vi "Steuerprogramm_ECD-HorstTest.vi"() -> ()   [LabVIEW 2017]
uses:
  <vilib>/FPGAPlugInAG/cRIO-9035/niLvFpga_Close_cRIO-9035.vi
  <vilib>/rvi/errors/niLvFpgaAdjustHostInterfaceError.vi
  <vilib>/Utility/error.llb/Error Cluster From Error Code.vi
  GVRefStrom.vi
  gvbooleschRT.vi
  GVMethodenwechsel.vi
  GVZeitenZyklen.vi
  GVaktuelleTDMS.vi
  GVChroms.vi
  GVMetavariablen.vi
  GVMWHorst.vi
  GVVentilposition.vi
  GVHK1Hz.vi
  GVZwangs.vi
  GVZwangsMPV.vi
  GVTrapsMachs.vi
  GVECDs.vi
  GVAIs.vi
  GVHeizenLH.vi
  GVHorstSP.vi
  GVProbenvol.vi
  <vilib>/rvi/interface/nirviCloseFPGA/nirviCloseFPGA.xnode
  FPGA Bitfiles/HAGAR-VECD_FPGATarget_FPGA-ProgrammECD_WS++LmW9gGg.lvbitx
  FPGA-Programm_ECD.vi
  <vilib>/rvi/interface/nirviReadWriteControl/nirviReadWriteControl.xnode
  <vilib>/rvi/interface/nirviMethod/nirviMethod.xnode
  <vilib>/rvi/errors/niLvFpgaMergeErrorWithErrorCode.vi
  <vilib>/FPGAPlugInAG/cRIO-9035/niLvFpga_WriteFifo_cRIO-9035.vi
  NiFpgaLv.dll
panel:
  out "Fehler ECD1alt":errorcluster caption="Fehler (Ausgang)"
  in  "Methode speichern":bool
  out "ZyklusNummernGesamt":i32[](array[numeric])
  in  "veränderte Methode benutzen":bool
  in  "Methode verändern":bool
  out "ZyklusNummern":i32[](array[numeric])
  out "Big Ben, Methodenzeit, Zykluszeit0, Zykluszeit1, Zykluszeit2A, Zykluszeit2B":i32[](array[numeric])
  in  "global stop RT":bool
  in  "Methode":i32(ring) items=["Bedingsmethode", "Startmethode", "Meßmodus", "Shut-up-Methode", "Test", "HAG2 1/2", "Startmethode", "HAG2 1/2 Aufwärmen", "LicorDruckProfil1", "LicorDruckProfil2", "LicorDruckProfil0", "LicorDruckProfil3"]
  in  "Registerkarte":T1(tab)
  out "SHOK?":bool[](array[boolean])
  out "schnelle Heizungen":string[](array[string])
  out "schnelle Heizungen":dbl[](array[numeric])
  out "HorstOK?":bool[](array[boolean])
  out "AIs3OK?":bool[](array[boolean])
  out "AIs1OK?":bool[](array[boolean])
  out "AIs1":dbl[](array[numeric])
  out "AIs1":string[](array[string])
  out "AIs2":string[](array[string])
  out "AIs3":string[](array[string])
  out "AIs2":dbl[](array[numeric])
  out "AIs3":dbl[](array[numeric])
  out "Metavariablen":string[](array[string])
  out "Metavariablen":dbl[](array[numeric])
  out "MWHorst":dbl[](array[numeric])
  out "HorstRegler":string[](array[string])
  out "AIs2OK?":bool[](array[boolean])
  out "Ventilposition":i32=1 min=1 max=6 step=1
  out "MVOK?":bool[](array[boolean])
  in  "MV-Vorgaben":dbl[](array[numeric])
  in  "MV-Festhalten":bool[](array[boolean])
  in  "LH-Gruppe":bool[](array[boolean])=[FALSE, FALSE, FALSE, FALSE, FALSE, FALSE, FALSE, FALSE, FALSE, FALSE, FALSE, FALSE]
  out "LangsameHeizungen":string[](array[string])
  out "Housekeeping1":cluster{dbl[], dbl[]}(graph)
  in  "Zeitachse1":i32(ring)=1 items=["Zykluszeit [s] Mod0", "Zykluszeit [s] Mod1", "Zykluszeit [s] Mod2A", "Zykluszeit [s] Mod2B"]
  in  "dargestellte Größe 1":i32(ring)=1 items=["T1-Trap1 [°C]", "T1-Trap2 [°C]", "T1-StirlingKühlkopf [°C]", "T1-PreCol1 [°C]", "T1-PreCol2 [°C]", "T1-MainCol1a [°C]", "T1-MainCol1b [°C]", "T1-MainCol2a [°C]", "T1-MainCol2b [°C]", "T1-Bronkhorst1a [°C]", "T1-Bronkhorst1b [°C]", "T1-Bronkhorst2a [°C]", "T1-Bronkhorst2b [°C]", "T1-2Pos1B [°C]", "T1-Spare9", "T1-2Pos1A [°C]", "T1-Spare10", "T1-TurboPump [°C]", "T1-StirlingPlatine [°C]", "T1-Spare5", "T1-Spare6", "T1-Spare7", "T1-Inlet [°C]", "F1-MFM1", "F1-MFM0D [mL]", "P1-HeliumHP [bara]", "P1-HeliumLP [bara]", "P1-PumpVordruck [mbara]", "TurboSpeed", "I1-MS-AC [A]", "I1-Trap1 [A]", "I1-Trap2 [A]", "T2-ECD1a", "T2-ECD1b", "T2-ECD2a", "T2-ECD2b", "T2-Col1a", "T2-Col1b", "T2-Col2a", "T2-Col2b", "T2-Spare1", "T2-Spare2", "T2-Oven_a", "T2-Oven_b", "T2-Spare3", "T2-Spare4", "T2-Spare5", "F2-MFM0", "F2-MFM2A", "F2-MFM2B", "P2-N2O_HP", "P2-N2O_LP", "P2-CO2_HP", "P2-CO2_LP", "AI-Spare1", "FL-MFM1000mL", "AI-Spare3", "AI-Spare4", "StirlingAlarm", "StirlingEmerg.", "AI-Spare7", "AI-Spare8", "AI-Spare9", "FL-MFM30mL", "T0-DC/DC5", "I0-24V_M0", "I0-48V_M1", "I0-24V_M1", "I0-28V_M2", "T0-Spare3", "T0-Spare2", "T0-Spare4", "T0-DC/DC7", "I0-20V_Laptop", "I0-28V_M1", "I0-24V_M2", "I0-12V_Licor", "T0-Spare1", "T0-Drier", "T0-Spare5", "F0-MFM0A [L]", "TL-Licor_a", "P0-Span-HP", "P0-spare1", "P0-Stickstoff-LP", "P0-Helium-LP", "P0-Cal-HP", "P0-P9Tavco[bar]", "F0-MFM0B [L]", "TL-Licor_b", "P0-Span-LP", "P0-spare2", "P0-Stickstoff-HP", "P0-Helium-HP", "P0-Cal-LP", "F0-MFM3", "TemperaturTrap1[°C]", "TemperaturTrap2[°C]", "TemperaturPreMach1[°C]", "TemperaturPreMach2[°C]", "TemperaturMainMach1[°C]", "TemperaturMainMach2[°C]", "PrC0 [bara]", "PrC0-Licor [bara]", "PrC1-Säule1 [bara]", "PrC1-Säule2 [bara]", "MFC1-Sample [ml/min]", "PrC1-BackFlush1 [bara]", "PrC1-BackFlush2 [bara]", "MFC1-Reaktant [l/min]", "MFC2A[ml/min]", "MFC2B[ml/min]", "MFC2C[ul/min]", "PrC2A[bara]", "MFC2D[ml/min]", "MFC2E[ml/min]", "PrC2B[bara]"]
  out "Housekeeping2":cluster{dbl[], dbl[]}(graph)
  in  "Zeitachse2":i32(ring)=1 items=["Zykluszeit [s] Mod0", "Zykluszeit [s] Mod1", "Zykluszeit [s] Mod2A", "Zykluszeit [s] Mod2B"]
  in  "dargestellte Größe 2":i32(ring)=1 items=["T1-Trap1 [°C]", "T1-Trap2 [°C]", "T1-StirlingKühlkopf [°C]", "T1-PreCol1 [°C]", "T1-PreCol2 [°C]", "T1-MainCol1a [°C]", "T1-MainCol1b [°C]", "T1-MainCol2a [°C]", "T1-MainCol2b [°C]", "T1-Bronkhorst1a [°C]", "T1-Bronkhorst1b [°C]", "T1-Bronkhorst2a [°C]", "T1-Bronkhorst2b [°C]", "T1-2Pos1B [°C]", "T1-Spare9", "T1-2Pos1A [°C]", "T1-Spare10", "T1-TurboPump [°C]", "T1-StirlingPlatine [°C]", "T1-Spare5", "T1-Spare6", "T1-Spare7", "T1-Inlet [°C]", "F1-MFM1", "F1-MFM0D [mL]", "P1-HeliumHP [bara]", "P1-HeliumLP [bara]", "P1-PumpVordruck [mbara]", "TurboSpeed", "I1-MS-AC [A]", "I1-Trap1 [A]", "I1-Trap2 [A]", "T2-ECD1a", "T2-ECD1b", "T2-ECD2a", "T2-ECD2b", "T2-Col1a", "T2-Col1b", "T2-Col2a", "T2-Col2b", "T2-Spare1", "T2-Spare2", "T2-Oven_a", "T2-Oven_b", "T2-Spare3", "T2-Spare4", "T2-Spare5", "F2-MFM0", "F2-MFM2A", "F2-MFM2B", "P2-N2O_HP", "P2-N2O_LP", "P2-CO2_HP", "P2-CO2_LP", "AI-Spare1", "FL-MFM1000mL", "AI-Spare3", "AI-Spare4", "StirlingAlarm", "StirlingEmerg.", "AI-Spare7", "AI-Spare8", "AI-Spare9", "FL-MFM30mL", "T0-DC/DC5", "I0-24V_M0", "I0-48V_M1", "I0-24V_M1", "I0-28V_M2", "T0-Spare3", "T0-Spare2", "T0-Spare4", "T0-DC/DC7", "I0-20V_Laptop", "I0-28V_M1", "I0-24V_M2", "I0-12V_Licor", "T0-Spare1", "T0-Drier", "T0-Spare5", "F0-MFM0A [L]", "TL-Licor_a", "P0-Span-HP", "P0-spare1", "P0-Stickstoff-LP", "P0-Helium-LP", "P0-Cal-HP", "P0-P9Tavco[bar]", "F0-MFM0B [L]", "TL-Licor_b", "P0-Span-LP", "P0-spare2", "P0-Stickstoff-HP", "P0-Helium-HP", "P0-Cal-LP", "F0-MFM3", "TemperaturTrap1[°C]", "TemperaturTrap2[°C]", "TemperaturPreMach1[°C]", "TemperaturPreMach2[°C]", "TemperaturMainMach1[°C]", "TemperaturMainMach2[°C]", "PrC0 [bara]", "PrC0-Licor [bara]", "PrC1-Säule1 [bara]", "PrC1-Säule2 [bara]", "MFC1-Sample [ml/min]", "PrC1-BackFlush1 [bara]", "PrC1-BackFlush2 [bara]", "MFC1-Reaktant [l/min]", "MFC2A[ml/min]", "MFC2B[ml/min]", "MFC2C[ul/min]", "PrC2A[bara]", "MFC2D[ml/min]", "MFC2E[ml/min]", "PrC2B[bara]"]
  out "Detektor 2":cluster{dbl[], dbl[]}[](graph)
  in  "Detektor":i32(ring) items=["ECD1", "ECD2"]
  in  "HK1YMin":dbl
  in  "HK1YMax":dbl=100.0
  in  "HK2YMin":dbl
  in  "HK2YMax":dbl=100.0
  in  "DetYMin":dbl
  in  "DetYMax":dbl=100.0
  in  "RefStromECD2":i16=2000 min=0 max=2500 step=1
  in  "RefStromECD1":i16=2000 min=0 max=2500 step=1
  out "schnelleAnzeige":cluster{dbl[], dbl[]}(graph)
  in  "TafelWischen!":bool
  in  "dargestellte Größe 3":i32(ring)=1 items=["TemperaturTrap1[°C]", "TemperaturTrap2[°C]", "TemperaturPreMach1[°C]", "TemperaturPreMach2[°C]", "TemperaturMainMach1[°C]", "TemperaturMainMach2[°C]", "PrC0 [bara]", "PrC0-Licor [bara]", "PrC1-Säule1 [bara]", "PrC1-Säule2 [bara]", "MFC1-Sample [ml/min]", "PrC1-BackFlush1 [bara]", "PrC1-BackFlush2 [bara]", "MFC1-Reaktant [l/min]", "MFC2A[ml/min]", "MFC2B[ml/min]", "MFC2C[ul/min]", "PrC2A[bara]", "MFC2D[ml/min]", "MFC2E[ml/min]", "PrC2B[bara]"]
  in  "An/Aus":bool
  out "TDMSwriteECD":errorcluster
  out "AIsFIFOread":errorcluster
  out "MWTrapsMachs":errorcluster
  out "TDMSwriteHK":errorcluster
  out "TDMScloseHK":errorcluster
  out "TDMSopenHK":errorcluster
  out "TDMScloseECD2":errorcluster
  out "TDMSopenECD2":errorcluster
  out "TDMScloseECD1":errorcluster
  out "TDMSopenECD1":errorcluster
  out "SerielleKomm.":errorcluster
  out "LH":errorcluster
  out "Zyklus":errorcluster
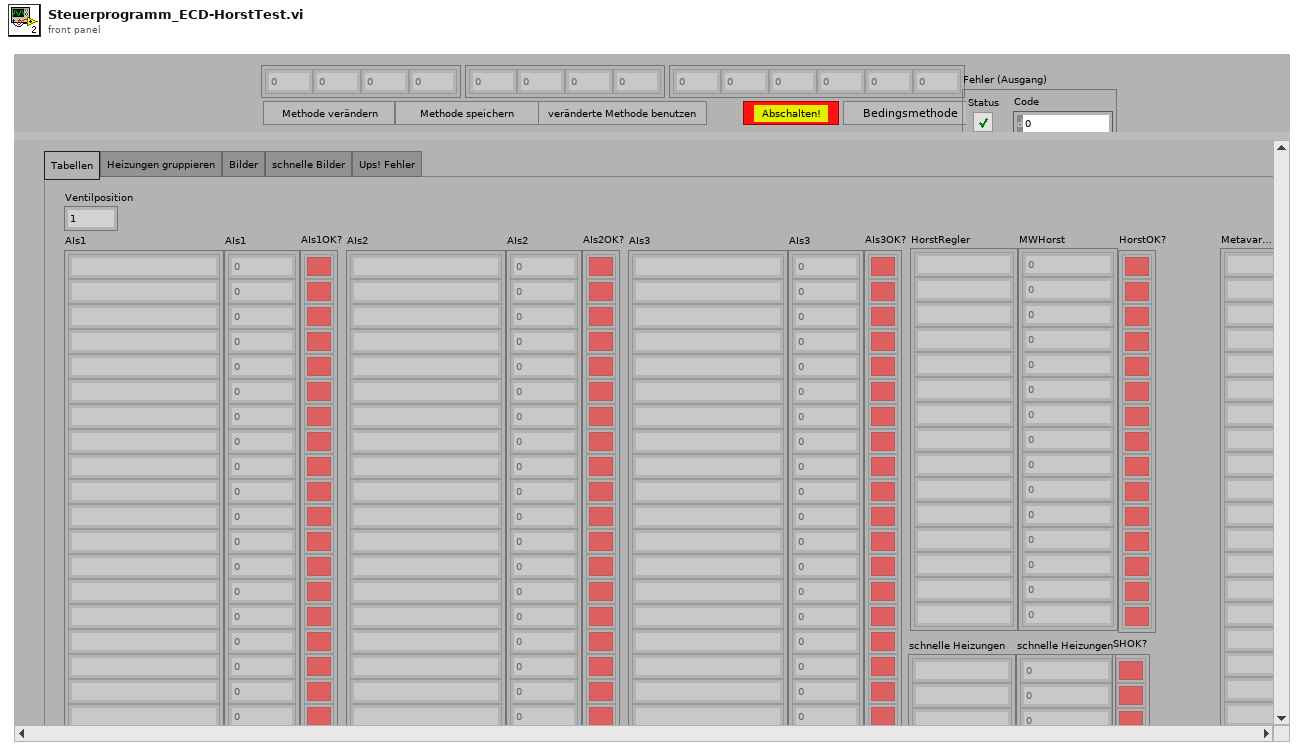
[diagram p1: front panel]
types:
  T1 = enum32{"Tabellen", "Heizungen gruppieren", "Bilder", "schnelle Bilder", "Ups! Fehler"}
  T2 = cluster{"DIOsMod0Nr":i32[], "DIOsMod1Nr":i32[], "DIOsMod2ANr":i32[], "DIOsMod2BNr":i32[], "AIsLH":i32[], "AnzahlRegler/Modul":i32[], "Regler für den Probenfluß":i32, "SPvorgebenMod0":string[], "SPvorgebenMod1":string[], "SPvorgebenMod2A":string[], "SPvorgebenMod2B":string[], "MWAntwortMod0":string[], "MWAntwortMod1":string[], "MWAntwortMod2A":string[], "MWAntwortMod2B":string[], "FaktorMod0":dbl[], "FaktorMod1":dbl[], "FaktorMod2A":dbl[], "FaktorMod2B":dbl[], "MWabfragenMod0":string[], "MWabfragenMod1":string[], "MWabfragenMod2A":string[], "MWabfragenMod2B":string[], "Modul1/AI koeff":dbl[][], "Modul2/AI koeff":dbl[][], "Modul3/AI koeff":dbl[][], "Traps/MachsKoeff T(R)":dbl[][], "Modul1/AIsNamen":string[], "Modul2/AIsNamen":string[], "Modul3/AIsNamen":string[], "DIOsMod0Name":string[], "DIOsMod1Name":string[], "DIOsMod2AName":string[], "DIOsMod2BName":string[], "ReglerNameMod0":string[], "ReglerNameMod1":string[], "ReglerNameMod2A":string[], "ReglerNameMod2B":string[], "Startmethode":i32, "Dateiordner Housekeeping":path, "Dateiname Housekeeping":string, "DateiordnerECD1":path, "DateinameECD1":string, "DateiordnerECD2":path, "DateinameECD2":string, "LangsameHeizungen":string[], "ModuleLH":i32[], "Metavariablen":string[], "Modul1/AI sicherer Bereich":dbl[][], "Modul2/AI sicherer Bereich":dbl[][], "Modul3/AI sicherer Bereich":dbl[][], "Traps/Machs sicherer Bereich":dbl[][], "ReglerMod0 sicherer Bereich":dbl[][], "ReglerMod1 sicherer Bereich":dbl[][], "ReglerMod2A sicherer Bereich":dbl[][], "ReglerMod2B sicherer Bereich":dbl[][], "Metavariablen grüner Bereich":dbl[][], "Traps/MachsKoeff R(U)":dbl[][], "LHGruppe":bool[]}
  T3 = cluster{"Zykluslängen [s]":dbl[], "ZeitpktDIOsMod0":dbl[], "ZeitpktDIOsMod1":dbl[], "ZeitpktDIOsMod2A":dbl[], "ZeitpktDIOsMod2B":dbl[], "DIOsSPMod0":bool[][], "DIOsSPMod1":bool[][], "DIOsSPMod2A":bool[][], "DIOsSPMod2B":bool[][], "Mod0HorstZeitpkt":dbl[], "Mod1HorstZeitpkt":dbl[], "Mod2AHorstZeitpkt":dbl[], "Mod2BHorstZeitpkt":dbl[], "HorstSPMod0":dbl[][], "HorstSPMod1":dbl[][], "HorstSPMod2A":dbl[][], "HorstSPMod2B":dbl[][], "LHSetpoints":dbl[], "LHHeizen?":bool[], "ZPktFPGABoolesch":dbl[], "FPGABoolesch":bool[][], "ZeitpktFPGAPID":dbl[], "FPGAPID":cluster{"d0":fxp<+/-,18,18>, "d1":fxp<+/-,21,21>}[][], "ZeitpktFPGAFixp":dbl[], dbl[][], "t_PreMach1":dbl[], "T_PreMach1":dbl[], "t_PreMach2":dbl[], "T_PreMach2":dbl[], "PIDs für \"träge\" Heizungen":cluster{"proportional gain (Kc)":dbl, "integral time (Ti, min)":dbl, "derivative time (Td, min)":dbl}[], "Zwangsbedingungen":dbl[][], "Dateien fürs MS schicken?":bool, "ZeitpunkteMPV":dbl[], "SPMPV":i32[], "ZeitpktMS-1":dbl, "ZeitpktMS-2":dbl, "Int.Start1":dbl, "Int.Stop1":dbl, "Int.Start2":dbl, "Int.Stop2":dbl, "Methodenname":string, "t_MainMach1":dbl[], "T_MainMach1":dbl[], "t_MainMach2":dbl[], "T_MainMach2":dbl[]}[]
  T4 = enum16{"open", "replace", "create", "open or create", "replace or create", "replace or create with confirmation"}
  T5 = cluster{"Zyklus1":i32, "Zeitachse1":i32, "dargestellte Größe 1":i32, "Zyklus2":i32, "Zeitachse2":i32, "dargestellte Größe 2":i32}
  T6 = cluster{"DIOsMod0Name":string[], "DIOsMod1Name":string[], "DIOsMod2AName":string[], "DIOsMod2BName":string[], "ReglerNameMod0":string[], "ReglerNameMod1":string[], "ReglerNameMod2A":string[], "ReglerNameMod2B":string[], "LangsameHeizungen":string[]}
  T7 = cluster{"Zykluslängen [s]":dbl[], "ZeitpktDIOsMod0":dbl[], "ZeitpktDIOsMod1":dbl[], "ZeitpktDIOsMod2A":dbl[], "ZeitpktDIOsMod2B":dbl[], "DIOsSPMod0":bool[][], "DIOsSPMod1":bool[][], "DIOsSPMod2A":bool[][], "DIOsSPMod2B":bool[][], "Mod0HorstZeitpkt":dbl[], "Mod1HorstZeitpkt":dbl[], "Mod2AHorstZeitpkt":dbl[], "Mod2BHorstZeitpkt":dbl[], "HorstSPMod0":dbl[][], "HorstSPMod1":dbl[][], "HorstSPMod2A":dbl[][], "HorstSPMod2B":dbl[][], "LHSetpoints":dbl[], "LHHeizen?":bool[], "ZPktFPGABoolesch":dbl[], "FPGABoolesch":bool[][], "ZeitpktFPGAPID":dbl[], "FPGAPID":cluster{"d0":fxp<+/-,18,18>, "d1":fxp<+/-,21,21>}[][], "ZeitpktFPGAFixp":dbl[], dbl[][], "t_PreMach1":dbl[], "T_PreMach1":dbl[], "t_PreMach2":dbl[], "T_PreMach2":dbl[], "PIDs für \"träge\" Heizungen":cluster{"proportional gain (Kc)":dbl, "integral time (Ti, min)":dbl, "derivative time (Td, min)":dbl}[], "Zwangsbedingungen":dbl[][], "Dateien fürs MS schicken?":bool, "ZeitpunkteMPV":dbl[], "SPMPV":i32[], "ZeitpktMS-1":dbl, "ZeitpktMS-2":dbl, "Int.Start1":dbl, "Int.Stop1":dbl, "Int.Start2":dbl, "Int.Stop2":dbl, "Methodenname":string, "t_MainMach1":dbl[], "T_MainMach1":dbl[], "t_MainMach2":dbl[], "T_MainMach2":dbl[]}
  T8 = cluster{"Modul1/AI sicherer Bereich":dbl[][], "Modul2/AI sicherer Bereich":dbl[][], "Modul3/AI sicherer Bereich":dbl[][], "Traps/Machs sicherer Bereich":dbl[][], dbl[][], "Metavariablen grüner Bereich":dbl[][]}
  T9 = cluster{"created path":path, "created path":path, "created path":path, "Dateiname Housekeeping":string, "DateinameECD1":string, "DateinameECD2":string, "tdms0":refnum<k34>, "tdms1":refnum<k34>, "tdms0":refnum<k34>, "tdms1":refnum<k34>, "tdms0":refnum<k34>, "tdms1":refnum<k34>}
  T10 = cluster{"d0":fxp<+/-,18,18>, "d1":fxp<+/-,21,21>}[][]
  T11 = cluster{"proportional gain (Kc)":dbl, "integral time (Ti, min)":dbl, "derivative time (Td, min)":dbl}[]
  T12 = cluster{cluster{"ZeitpktDIOsMod2B":dbl[]}[], cluster{"DIOsSPMod2B":bool[][]}[], cluster{"Mod2BHorstZeitpkt":dbl[]}[], cluster{"HorstSPMod2B":dbl[][]}[], "LHHeizen?":bool[], "ZPktFPGABoolesch":dbl[], "FPGABoolesch":bool[][], "ZeitpktFPGAPID":dbl[], "FPGAPID":cluster{"d0":fxp<+/-,18,18>, "d1":fxp<+/-,21,21>}[][], "ZeitpktFPGAFixp":dbl[], dbl[][], "t_PreMach1":dbl[], "T_PreMach1":dbl[], "t_PreMach2":dbl[], "T_PreMach2":dbl[], "ZeitpunkteMPV":dbl[], "SPMPV":i32[], "t_MainMach1":dbl[], "T_MainMach1":dbl[], "t_MainMach2":dbl[], "T_MainMach2":dbl[]}
  T13 = cluster{"Zykluslängen [s]":dbl[], "ZeitpktDIOsMod0":dbl[], "ZeitpktDIOsMod1":dbl[], "ZeitpktDIOsMod2A":dbl[], "ZeitpktDIOsMod2B":dbl[], "DIOsSPMod0":bool[][], "DIOsSPMod1":bool[][], "DIOsSPMod2A":bool[][], "DIOsSPMod2B":bool[][], "Mod0HorstZeitpkt":dbl[], "Mod1HorstZeitpkt":dbl[], "Mod2AHorstZeitpkt":dbl[], "Mod2BHorstZeitpkt":dbl[], "HorstSPMod0":dbl[][], "HorstSPMod1":dbl[][], "HorstSPMod2A":dbl[][], "HorstSPMod2B":dbl[][], "LangsameHeizungenSP":dbl[], "LHHeizen?":bool[], "ZPktFPGABoolesch":dbl[], "FPGABoolesch":bool[][], "ZeitpktFPGAPID":dbl[], "FPGAPID":cluster{"d0":fxp<+/-,18,18>, "d1":fxp<+/-,21,21>}[][], "ZeitpktFPGAFixp":dbl[], "FPGAFixp":dbl[][], "t_PreMach1":dbl[], "T_PreMach1":dbl[], "t_PreMach2":dbl[], "T_PreMach2":dbl[], "PIDs für \"träge\" Heizungen":cluster{"proportional gain (Kc)":dbl, "integral time (Ti, min)":dbl, "derivative time (Td, min)":dbl}[], "Zwangsbedingungen":dbl[][], "MS-Daten?":bool, "ZeitpunkteMPV":dbl[], "SetpointMPV":i32[], "ZeitpktMS-1":dbl, "ZeitpktMS-2":dbl, "Int.Start1":dbl, "Int.Stop1":dbl, "Int.Start2":dbl, "Int.Stop2":dbl, "Methodenname":string, "t_MainMach1":dbl[], "T_MainMach1":dbl[], "t_MainMach2":dbl[], "T_MainMach2":dbl[]}
  T14 = cluster{"ZyklusNummern":i32[], "ZeilennummernDIOs":i32[], "ZwangsDIO?":cluster{bool[]}[], "ZeilennummernHorst":i32[], "ZwangsHorst?":cluster{bool[]}[], "ZeileFPGABoolesch":i32, "ZwangsFPGABoolesch?":bool[], "ZeileFPGAPID":i32, "ZeileFPGAFixp":i32, "ZeilePreMach1":i32, "ZeilePreMach2":i32, "ZeilennummerMPV":i32, "ZeileMainMach1":i32, "ZeileMainMach2":i32, "ZwangsMPV?":bool}
  T15 = cluster{"ZyklusNummern":i32[], i32[], "ZwangsDIO?":cluster{bool[]}[], i32[], "ZwangsHorst?":cluster{bool[]}[], i32, "ZwangsFPGABoolesch?":bool[], i32, i32, "ZeileMach":i32, "ZeileMach":i32, i32, "ZeileMach":i32, "ZeileMach":i32, "ZwangsMPV?":bool}
  T16 = cluster{string[], string[], string[], dbl[], dbl[], dbl[]}
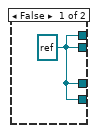
[diagram p2: hidden frame]
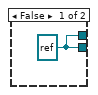
[diagram p3: hidden frame]
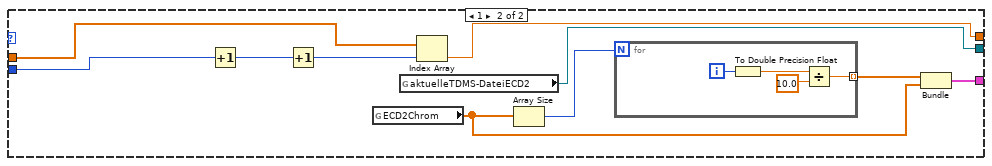
[diagram p13: hidden frame]
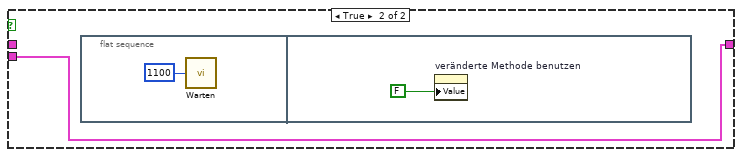
[diagram p14: hidden frame]
diagram:
  n1 = Open/Create/Replace File(file path (use dialog)=path "c:/einstellungen.pery" ("Datei (Dialog verwenden)"), operation (0:open)=T4."open" ("Operation (0:Öffnen)")) -> (refnum out=w15:refnum<file>)  [unwired: 4 in, 2 out]
  n2 = Open/Create/Replace File(file path (use dialog)=path "c:/methoden.pery" ("Datei (Dialog verwenden)"), operation (0:open)=T4."open" ("Operation (0:Öffnen)")) -> (refnum out=w10:refnum<file>)  [unwired: 4 in, 2 out]
  n3 = Read from Binary File(5:T2 {"DIOsMod0Nr"=[], "DIOsMod1Nr"=[], "DIOsMod2ANr"=[], "DIOsMod2BNr"=[], "AIsLH"=[], "AnzahlRegler/Modul"=[], "Regler für den Probenfluß"=0, "SPvorgebenMod0"=[], "SPvorgebenMod1"=[], "SPvorgebenMod2A"=[], "SPvorgebenMod2B"=[], "MWAntwortMod0"=[], "MWAntwortMod1"=[], "MWAntwortMod2A"=[], "MWAntwortMod2B"=[], "FaktorMod0"=[], "FaktorMod1"=[], "FaktorMod2A"=[], "FaktorMod2B"=[], "MWabfragenMod0"=[], "MWabfragenMod1"=[], "MWabfragenMod2A"=[], "MWabfragenMod2B"=[], "Modul1/AI koeff"=[], "Modul2/AI koeff"=[], "Modul3/AI koeff"=[], "Traps/MachsKoeff T(R)"=[], "Modul1/AIsNamen"=[], "Modul2/AIsNamen"=[], "Modul3/AIsNamen"=[], "DIOsMod0Name"=[], "DIOsMod1Name"=[], "DIOsMod2AName"=[], "DIOsMod2BName"=[], "ReglerNameMod0"=[], "ReglerNameMod1"=[], "ReglerNameMod2A"=[], "ReglerNameMod2B"=[], "Startmethode"=0, "Dateiordner Housekeeping"=path "", "Dateiname Housekeeping"="", "DateiordnerECD1"=path "", "DateinameECD1"="", "DateiordnerECD2"=path "", "DateinameECD2"="", "LangsameHeizungen"=[], "ModuleLH"=[], "Metavariablen"=[], "Modul1/AI sicherer Bereich"=[], "Modul2/AI sicherer Bereich"=[], "Modul3/AI sicherer Bereich"=[], "Traps/Machs sicherer Bereich"=[], "ReglerMod0 sicherer Bereich"=[], "ReglerMod1 sicherer Bereich"=[], "ReglerMod2A sicherer Bereich"=[], "ReglerMod2B sicherer Bereich"=[], "Metavariablen grüner Bereich"=[], "Traps/MachsKoeff R(U)"=[], "LHGruppe"=[]} ("Ausgangs-Cluster"), 11:w15) -> (2:w13:T2, 3:w14:refnum<file>)  [unwired: 4 in, 2 out]
  n4 = Read from Binary File(5:T3 [], 11:w10) -> (2:w8:T3, 3:w9:refnum<file>)  [unwired: 4 in, 2 out]
  n5 = Close File(refnum=w14) -> ()  [unwired: 1 in, 2 out]
  n6 = Close File(refnum=w9) -> ()  [unwired: 1 in, 2 out]
  n7 = flat-sequence {
    tunnel: [w61] -> w43
    tunnel: [w125] -> w42
    tunnel: [w65] -> w40
    tunnel: [w256] -> w39
    tunnel: [w258] -> w38
    tunnel: [w250] -> w37
    tunnel: [w257] -> w36
    tunnel: [w182] -> w35
    tunnel: [w249] -> w34
    tunnel: [w248] -> w33
    tunnel: [w242] -> w32
    tunnel: [w185] -> w31
    tunnel: [w159] -> w30
    tunnel: [w255] -> w29
    tunnel: [w247] -> w28
    tunnel: [w246] -> w27
    tunnel: [w238] -> w26
    tunnel: [w237] -> w25
    tunnel: [w236] -> w24
    tunnel: [w235] -> w23
    tunnel: [w234] -> w22
    tunnel: [w233] -> w21
    tunnel: [w230] -> w20
    tunnel: [w212] -> w19
    tunnel: w13 -> [w104]
    tunnel: [w211] -> w18
    tunnel: w8 -> [w126]
    tunnel: [w125] -> w7
    tunnel: [w104] -> w6
    tunnel: [w73] -> w5
    tunnel: [w56] -> w2
    tunnel: [w48] -> w1
    tunnel: w43 -> [w323]
    tunnel: w42 -> [w392]
    tunnel: [w323] -> w41
    tunnel: w40 -> [_]
    tunnel: w39 -> [w351]
    tunnel: w38 -> [w294]
    tunnel: w37 -> [w352]
    tunnel: w36 -> [w350]
    tunnel: w35 -> [w327]
    tunnel: w34 -> [w322]
    tunnel: w33 -> [w319]
    tunnel: w32 -> [w316]
    tunnel: w31 -> [w317]
    tunnel: w30 -> [w320]
    tunnel: w29 -> [w390]
    tunnel: w28 -> [w325]
    tunnel: w27 -> [w391]
    tunnel: w26 -> [w302]
    tunnel: w25 -> [w301]
    tunnel: w24 -> [w300]
    tunnel: w23 -> [w388]
    tunnel: w22 -> [w387]
    tunnel: w21 -> [w386]
    tunnel: w20 -> [w342]
    tunnel: w19 -> [w326]
    tunnel: w18 -> [w315]
    tunnel: w8 -> [w314]
    tunnel: w7 -> [w312]
    tunnel: w6 -> [_]
    tunnel: w5 -> [w295]
    tunnel: w2 -> [w292]
    tunnel: w1 -> [w291]
    tunnel: w41 -> [w1042]
    frame #0 {
      w55 = i16 2000 ("RefStromECD1")
      w127 = TRUE
      w141 = 0.0 ("Probenvol.1")
      w148 = dbl[] [-1.0] ("ECD1MW")
      w149 = FALSE ("ECD1Empfangen?")
      w140 = string[] ["TemperaturTrap1[°C]", "TemperaturTrap2[°C]", "TemperaturPreMach1[°C]", "TemperaturPreMach2[°C]", "TemperaturMainMach1[°C]", "TemperaturMainMach2[°C]"]
      w253 = string[] ["Big Ben [s]", "Methodenzeit [s]", "Zykluszeit [s] Mod0", "Zykluszeit [s] Mod1", "Zykluszeit [s] Mod2A", "Zykluszeit [s] Mod2B"]
      w243 = FALSE ("Undefinierte Werte möglich")
      w244 = FALSE ("global stop RT")
      n8 = for {
        tunnel: [w286] -> w251 mode=indexing
        tunnel: w126 -> [w287] mode=indexing
        n9 = Unbundle(w287) -> ("Methodenname"=w286:string)  [unwired: 44 out]
      }
      n10 = Unbundle(w104) -> ("DIOsMod0Nr"=w169:i32[], "DIOsMod1Nr"=w168:i32[], "DIOsMod2ANr"=w167:i32[], "DIOsMod2BNr"=w166:i32[], "AIsLH"=w156:i32[], "AnzahlRegler/Modul"=w159:i32[], "Regler für den Probenfluß"=w211:i32, "SPvorgebenMod0"=w210:string[], "SPvorgebenMod1"=w209:string[], "SPvorgebenMod2A"=w208:string[], "SPvorgebenMod2B"=w207:string[], "MWAntwortMod0"=w206:string[], "MWAntwortMod1"=w205:string[], "MWAntwortMod2A"=w57:string[], "MWAntwortMod2B"=w58:string[], "FaktorMod0"=w204:dbl[], "FaktorMod1"=w203:dbl[], "FaktorMod2A"=w202:dbl[], "FaktorMod2B"=w201:dbl[], "MWabfragenMod0"=w200:string[], "MWabfragenMod1"=w199:string[], "MWabfragenMod2A"=w198:string[], "MWabfragenMod2B"=w197:string[], "Modul1/AI koeff"=w196:dbl[][], "Modul2/AI koeff"=w195:dbl[][], "Modul3/AI koeff"=w194:dbl[][], "Traps/MachsKoeff T(R)"=w193:dbl[][], "Modul1/AIsNamen"=w192:string[], "Modul2/AIsNamen"=w191:string[], "Modul3/AIsNamen"=w190:string[], "DIOsMod0Name"=w102:string[], "DIOsMod1Name"=w103:string[], "DIOsMod2AName"=w101:string[], "DIOsMod2BName"=w100:string[], "ReglerNameMod0"=w118:string[], "ReglerNameMod1"=w117:string[], "ReglerNameMod2A"=w116:string[], "ReglerNameMod2B"=w115:string[], "Startmethode"=w125:i32, "Dateiordner Housekeeping"=w99:path, "Dateiname Housekeeping"=w189:string, "DateiordnerECD1"=w54:path, "DateinameECD1"=w188:string, "DateiordnerECD2"=w112:path, "DateinameECD2"=w187:string, "LangsameHeizungen"=w186:string[], "ModuleLH"=w181:i32[], "Metavariablen"=w120:string[], "Modul1/AI sicherer Bereich"=w77:dbl[][], "Modul2/AI sicherer Bereich"=w76:dbl[][], "Modul3/AI sicherer Bereich"=w75:dbl[][], "Traps/Machs sicherer Bereich"=w74:dbl[][], "ReglerMod0 sicherer Bereich"=w72:dbl[][], "ReglerMod1 sicherer Bereich"=w71:dbl[][], "ReglerMod2A sicherer Bereich"=w70:dbl[][], "ReglerMod2B sicherer Bereich"=w69:dbl[][], "Metavariablen grüner Bereich"=w67:dbl[][], "LHGruppe"=w60:bool[])  [unwired: 1 out]
      "Metavariablen" <- w120
      "LangsameHeizungen" <- w186
      n11 = Initialize Array(0, 4 ("Dimension")) -> (w142:i32[])
      n12 = Initialize Array(0.0 ("Element"), 6 ("Dimension")) -> (w145:dbl[])
      n13 = global write "GVMethodenwechsel.vi" "Methodenwechsel?"(FALSE ("Methodenwechsel?")) -> ()
      n14 = global write "GVRefStrom.vi" "RefStromECD2"(w55) -> ()
      n15 = global write "GVRefStrom.vi" "RefStromECD1"(w55) -> ()
      n16 = property on="dargestellte Größe 2" class="Ring (strikt)"("AllowUndefVals"=w243) -> ()  [unwired: 2 in, 2 out]
      n17 = property on="Zeitachse2" class="Ring (strikt)"("AllowUndefVals"=w243) -> ()  [unwired: 2 in, 2 out]
      n18 = property on="Zeitachse1" class="Ring (strikt)"("AllowUndefVals"=w243) -> ()  [unwired: 2 in, 2 out]
      n19 = property on="dargestellte Größe 1" class="Ring (strikt)"("AllowUndefVals"=w243) -> ()  [unwired: 2 in, 2 out]
      n20 = property on="Methode" class="Ring (strikt)"("AllowUndefVals"=w243) -> ()  [unwired: 2 in, 2 out]
      n21 = global write "GVProbenvol.vi" "Probenvol.1"(w141) -> ()
      n22 = global write "GVProbenvol.vi" "Probenvol.2"(w141) -> ()
      n23 = global write "GVECDs.vi" "ECD1MW"(w148) -> ()
      n24 = global write "GVECDs.vi" "ECD2MW"(w148) -> ()
      n25 = global write "GVECDs.vi" "ECD1Empfangen?"(w149) -> ()
      n26 = global write "GVECDs.vi" "ECD2Empfangen?"(w149) -> ()
      n27 = local write "global stop RT"(w244) -> ()
      n28 = global write "gvbooleschRT.vi" "global stop RT"(w244) -> ()
      n29 = global write "GVZeitenZyklen.vi" "ZyklusNummern"(w142) -> ()
      n30 = global write "GVZeitenZyklen.vi" "ZyklusNummernGesamt"(w142) -> ()
      n31 = global write "GVZeitenZyklen.vi" "Big Ben, Methodenzeit, Zykluszeit0, Zykluszeit1, Zykluszeit2A, Zykluszeit2B"(w145) -> ()
      n32 = property on="Methode" class="Ring (strikt)"("Value"=w125) -> ()  [unwired: 2 in, 2 out]
      n33 = Build Array (concatenate)(w57, w58) -> (w56:string[])
      n34 = Initialize Array(-1.0 ("Element"), 6 ("Dimension")) -> (w152:dbl[])
      n35 = Initialize Array(FALSE, 10 ("Dimension")) -> (w160:bool[])
      n36 = Initialize Array(-1.0 ("Element"), 96 ("Dimension")) -> (w153:dbl[])
      n37 = local write "LH-Gruppe"(w60) -> ()
      n38 = global write "GVZwangs.vi" "ZwangsFPGABoolesch!"(w160) -> ()
      n39 = global write "GVZwangs.vi" "ZwangsFPGABoolesch?"(w160) -> ()
      n40 = global write "GVTrapsMachs.vi" "Traps/Machs"(w152) -> ()
      n41 = global write "GVAIs.vi" "AIs"(w153) -> ()
      n42 = for {
        tunnel: w159 -> [w264] mode=indexing
        tunnel: [w261] -> w158 mode=indexing
        tunnel: [w259] -> w157 mode=indexing
        n43 = Initialize Array(0.0 ("Element"), w264) -> (w262:dbl[])
        n44 = Initialize Array(FALSE, w264) -> (w260:bool[])
        n45 = Bundle(w262) -> (w261:cluster{dbl[]})  [unwired: 1 in]
        n46 = Bundle(w260) -> (w259:cluster{bool[]})  [unwired: 1 in]
      }
      n47 = Bundle("DIOsMod0Name"=w102, "DIOsMod1Name"=w103, "DIOsMod2AName"=w101, "DIOsMod2BName"=w100, "ReglerNameMod0"=w118, "ReglerNameMod1"=w117, "ReglerNameMod2A"=w116, "ReglerNameMod2B"=w115, "LangsameHeizungen"=w186) -> (w246:T6)  [unwired: 1 in]
      n48 = Build Array (concatenate)(w118, w117, w116, w115) -> (w139:string[])
      n49 = Build Array (concatenate)(w206, w205, w57, w58) -> (w257:string[])
      n50 = Build Array (concatenate)(w210, w209, w208, w207) -> (w258:string[])
      n51 = Build Array (concatenate)(w204, w203, w202, w201) -> (w250:dbl[])
      n52 = Build Array (concatenate)(w200, w199, w198, w197) -> (w256:string[])
      n53 = Build Array (concatenate)(w118, w117, w116, w115) -> (→"HorstRegler":string[])
      n54 = Build Array (concatenate)(w72, w71, w70, w69) -> (w68:dbl[][])
      n55 = Array Size(array=w120) -> (size(s)=w47:i32)
      n56 = Build Array(w169, w168, w167, w166) -> (w165:i32[][])
      n57 = Array Size(array=w186) -> (size(s)=w185:i32)
      n58 = Add Array Elements(numeric array=w159) -> (sum=w242:i32)
      n59 = Array Size(array=w156) -> (size(s)=w155:i32)
      n60 = Index Array(array=w126, index=w125) -> (element=w124:T7)
      n61 = Add Array Elements(numeric array=w159) -> (sum=w171:i32)
      n62 = Decrement(x=w181) -> (x-1=w180:i32[])
      n63 = Build Cluster Array(w169, w168, w167, w166) -> (w249:cluster{"DIOsMod2BNr":i32[]}[])
      n64 = Build Array (concatenate)(w192, w191, w190) -> (w59:string[])
      n65 = Index Array(array=w193, index (col)=2 ("Deaktivierter Index (Spalte)")) -> (element=w238:dbl[])  [unwired: 1 in]
      n66 = Index Array(array=w193, index (col)=0 ("Deaktivierter Index (Spalte)")) -> (element=w236:dbl[])  [unwired: 1 in]
      n67 = Index Array(array=w193, index (col)=1 ("Deaktivierter Index (Spalte)")) -> (element=w237:dbl[])  [unwired: 1 in]
      n68 = Concatenate Strings("?SE0,SETP,2000" ("string"), "\n") -> (w79:string)
      n69 = Concatenate Strings("?SE0,SETP,2000" ("string"), "\n") -> (w86:string)
      n70 = for {
        tunnel: w249 -> [w289] mode=indexing
        tunnel: [w290] -> w248 mode=indexing
        n71 = Unbundle(w289) -> ("DIOsMod2BNr"=w288:i32[])
        n72 = Array Size(array=w288) -> (size(s)=w290:i32)
      }
      n73 = property on="Methode" class="Ring (strikt)"("Strings []"=w251) -> ()  [unwired: 2 in, 2 out]
      n74 = Bundle("Modul1/AI sicherer Bereich"=w77, "Modul2/AI sicherer Bereich"=w76, "Modul3/AI sicherer Bereich"=w75, "Traps/Machs sicherer Bereich"=w74, w68, "Metavariablen grüner Bereich"=w67) -> (w73:T8)  [unwired: 1 in]
      n75 = Build Array (concatenate)(w153, w152) -> (w151:dbl[])
      n76 = Array Size(array=w165) -> (size(s)=w164:i32[])
      n77 = Unbundle(w124) -> ("SPMPV"=w123:i32[])  [unwired: 44 out]
      n78 = Open/Create/Replace File(file path (use dialog)=path "c:/fromcriordy.txt" ("Dateipfad (Dialog verwenden)"), operation (0:open)=T4."replace or create" ("Operation (0:Öffnen)")) -> (refnum out=w215:refnum<file>, error out=w216:errorcluster)  [unwired: 4 in, 1 out]
      n79 = Initialize Array(FALSE, w47) -> (w45:bool[])
      n80 = Initialize Array(0.0 ("element"), w47) -> (w44:dbl[])
      n81 = Initialize Array(0.0 ("Element"), w171) -> (w170:dbl[])
      n82 = Get Date/Time In Seconds() -> (seconds since 1Jan1904=w113:timestamp)
      n83 = Initialize Array(FALSE, w155) -> (w150:bool[])
      n84 = Multiply(x=w180, y=32) -> (x*y=w183:i32[])
      n85 = Initialize Array(-1.0, w171) -> (w173:dbl[])
      n86 = Array Subset(array=w59, index=32 ("Index"), length=32 ("Länge")) -> (→"AIs2":string[])
      n87 = Array Subset(array=w59, index=0 ("Index"), length=32 ("Länge")) -> (→"AIs1":string[])
      n88 = Array Subset(array=w59, index=64 ("Index"), length=32 ("Länge")) -> (→"AIs3":string[])
      n89 = global write "GVMetavariablen.vi" "MV-Festhalten"(w45) -> ()
      n90 = global write "GVMetavariablen.vi" "MV-Vorgaben"(w44) -> ()
      n91 = global write "GVHK1Hz.vi" "Mod1Mod2Mod3/AITrapsMachs1Hz"(w151) -> ()
      n92 = global write "GVMetavariablen.vi" "Metavariablen"(w44) -> ()
      n93 = global write "GVHeizenLH.vi" "Heizen?LH"(w150) -> ()
      n94 = global write "GVZwangs.vi" "ZwangsLangsameHeizungenAn!"(w150) -> ()
      n95 = for {
        tunnel: w164 -> [w269] mode=indexing
        tunnel: [w266] -> w163 mode=indexing
        n96 = Initialize Array(FALSE, w269) -> (w267:bool[])
        n97 = Bundle(w267) -> (w266:cluster{bool[]})  [unwired: 1 in]
      }
      n98 = global write "GVHorstSP.vi" "HorstSP"(w170) -> ()
      n99 = global write "GVZwangs.vi" "ZwangsLangsameHeizungenAn?"(w150) -> ()
      n100 = local write "MV-Festhalten"(w45) -> ()
      n101 = Add(x=w183, y=w156) -> (x+y=w182:i32[])
      n102 = Close File(refnum=w215, error in=w216) -> (path=w247:path)  [unwired: 1 out]
      n103 = Format Date/Time String(time format string (%c)="%Y-%m-%d--%H-%M" ("Zeitformatierungs-String (%c)"), seconds (now)=w113) -> (date/time string=w52:string)  [unwired: 1 in]
      n104 = String To Byte Array(string=w79) -> (unsigned byte array=w81:u8[])
      n105 = String To Byte Array(string=w86) -> (unsigned byte array=w91:u8[])
      n106 = Index Array(array=w123, index=0) -> (element=w121:i32)
      n107 = call "FPGA-Start_ECD.vi"() -> ("error out"=w65:errorcluster, "FPGA-VI-Referenz (Ausgang)"=w64:refnum<k20>)  [unwired: 2 in]
      n108 = local write "MV-Vorgaben"(w44) -> ()
      n109 = global write "GVMWHorst.vi" "MWHorst"(w173) -> ()
      n110 = global write "GVVentilposition.vi" "Ventilposition"(w121) -> ()
      n111 = Build Array (concatenate)(string[] ["Jahr", "Monat", "Tag", "Stunde", "Minute", "Sekunde"] ("Array"), string[] ["Datei Nr.", "Methode Nr.", "Zyklusnr. Mod0", "Zyklusnr. Mod1", "Zyklusnr. Mod2A", "Zyklusnr. Mod2B"], w253, w59, w140, w139, "Probenvolumen1", "Probenvolumen2", "Ventilposition" ("element"), string[] ["CPU Total", "CPU Time critical", "CPU Timed Structures", "CPU High", "CPU Above normal", "CPU Normal", "CPU Background", "CPU Idle", "CPU ISR", "Memory", "SekundenTotalBrutal"]) -> (w255:string[])
      n112 = Build Array (concatenate)(w140, w139) -> (w138:string[])
      n113 = Build Array (concatenate)(w59, w140, w139) -> (w137:string[])
      n114 = Join Numbers(hi=w81, lo=u8 5) -> ((hi.lo)=w78:u16[])
      n115 = Join Numbers(hi=w91, lo=u8 6) -> ((hi.lo)=w89:u16[])
      n116 = Split 1D Array(array=w253, index=2 ("Index")) -> (second subarray=w245:string[])  [unwired: 1 out]
      n117 = Concatenate Strings("HK " ("String"), w52) -> (w96:string)
      n118 = Concatenate Strings("ECD1 " ("String"), w52) -> (w95:string)
      n119 = Concatenate Strings("ECD2 " ("String"), w52) -> (w93:string)
      n120 = property on="dargestellte Größe 1" class="Ring (strikt)"("Strings []"=w137) -> ()  [unwired: 2 in, 2 out]
      n121 = global write "GVZwangs.vi" "ZwangsHorst!"(w158) -> ()
      n122 = global write "GVZwangs.vi" "ZwangsHorst?"(w157) -> ()
      n123 = xnode "Invoke Method"("FPGA-VI-Referenz (Eingang)"=w64, "Daten"=w78) -> ("FPGA-VI-Referenz (Ausgang)"=w84:refnum<k20>)  [unwired: 2 in, 2 out]
      n124 = property on="dargestellte Größe 2" class="Ring (strikt)"("Strings []"=w137) -> ()  [unwired: 2 in, 2 out]
      n125 = property on="dargestellte Größe 3" class="Ring (strikt)"("Strings []"=w138) -> ()  [unwired: 2 in, 2 out]
      n126 = property on="Zeitachse2" class="Ring (strikt)"("Strings []"=w245) -> ()  [unwired: 2 in, 2 out]
      n127 = property on="Zeitachse1" class="Ring (strikt)"("Strings []"=w245) -> ()  [unwired: 2 in, 2 out]
      n128 = Concatenate Strings("ECD1alt" ("String"), w52) -> (w50:string)
      n129 = xnode "Invoke Method"("FPGA-VI-Referenz (Eingang)"=w84, "Daten"=w89) -> ("FPGA-VI-Referenz (Ausgang)"=w63:refnum<k20>)  [unwired: 2 in, 2 out]
      n130 = Build Path(base path=w99, name or relative path=w96) -> (appended path=w107:path)
      n131 = Build Path(base path=w54, name or relative path=w95) -> (appended path=w109:path)
      n132 = Build Path(base path=w112, name or relative path=w93) -> (appended path=w111:path)
      n133 = Build Path(base path=w54, name or relative path=w50) -> (appended path=w49:path)
      n134 = Create Folder(path (use dialog)=w49) -> (created path=w48:path)  [unwired: 2 in, 2 out]
      n135 = global write "GVZwangs.vi" "ZwangsDIO!"(w163) -> ()
      n136 = global write "GVZwangs.vi" "ZwangsDIO?"(w163) -> ()
      n137 = call "MPVSenden_ECD.vi"("Ventilposition"=0, "FPGA-VI-Referenz"=w63) -> ("FPGA-VI-Referenz (Ausgang)"=w61:refnum<k20>)  [unwired: 1 in, 2 out]
      n138 = Create Folder(path (use dialog)=w107) -> (created path=w106:path)  [unwired: 2 in, 2 out]
      n139 = Create Folder(path (use dialog)=w109) -> (created path=w108:path)  [unwired: 2 in, 2 out]
      n140 = Create Folder(path (use dialog)=w111) -> (created path=w110:path)  [unwired: 2 in, 2 out]
      n141 = case shown="True" w127 {
        tunnel: [w280 w285] -> w229
        tunnel: [w280 w284] -> w228
        tunnel: w106 -> [_ w283]
        tunnel: w189 -> [_ w282]
        tunnel: w125 -> [_ w281]
        frame False {
          w280 = refnum<k34> refnum ("tdms1")
        }
        frame True {
          n142 = call "TDMS0.vi"("Startmethode"=w281, "Dateiname"=w282, "Dateiordner"=w283) -> ("tdms1"=w284:refnum<k34>, "tdms0"=w285:refnum<k34>)
          n143 = global write "GVaktuelleTDMS.vi" "aktuelleTDMS-DateiHK"(w285) -> ()
        }
      }
      n144 = case shown="True" w127 {
        tunnel: [w270 w279] -> w227
        tunnel: [w270 w278] -> w226
        tunnel: [w270 w277] -> w225
        tunnel: [w270 w276] -> w224
        tunnel: w108 -> [_ w275]
        tunnel: w188 -> [_ w274]
        tunnel: w110 -> [_ w273]
        tunnel: w187 -> [_ w272]
        tunnel: w125 -> [_ w271]
        frame False {
          w270 = refnum<k34> refnum ("tdms0")
        }
        frame True {
          n145 = call "TDMS0.vi"("Startmethode"=w271, "Dateiname"=w274, "Dateiordner"=w275) -> ("tdms1"=w278:refnum<k34>, "tdms0"=w279:refnum<k34>)
          n146 = call "TDMS0.vi"("Startmethode"=w271, "Dateiname"=w272, "Dateiordner"=w273) -> ("tdms1"=w276:refnum<k34>, "tdms0"=w277:refnum<k34>)
          n147 = global write "GVaktuelleTDMS.vi" "aktuelleTDMS-DateiECD1"(w279) -> ()
          n148 = global write "GVaktuelleTDMS.vi" "aktuelleTDMS-DateiECD2"(w277) -> ()
        }
      }
      n149 = Open/Create/Replace File(file path (use dialog)=path "c:/fromcriocmd.txt" ("Pfad MS-Datei CRIO"), operation (0:open)=T4."replace or create" ("Operation (0:Öffnen)")) -> (refnum out=w221:refnum<file>, error out=w220:errorcluster)  [unwired: 4 in, 1 out]
      n150 = Write to Text File(file (use dialog)=w221, text="time=yyyymmddhhmmss\ncycle=005\ninfo=1234567890123456789012345678901234567890123456789012345678901234567890123456789012345678901234567890\nlength=100\ncmd=cycle" ("Text0 MS-Datei"), error in=w220) -> (refnum out=w218:refnum<file>, error out=w217:errorcluster)  [unwired: 1 in, 1 out]
      n151 = Bundle("created path"=w106, "created path"=w108, "created path"=w110, "Dateiname Housekeeping"=w189, "DateinameECD1"=w188, "DateinameECD2"=w187, "tdms0"=w229, "tdms1"=w228, "tdms0"=w227, "tdms1"=w226, "tdms0"=w225, "tdms1"=w224) -> (w230:T9)  [unwired: 1 in]
      n152 = call "AIKoeffSortieren.vi"("Modul3/AI koeff"=w194, "Modul2/AI koeff"=w195, "Modul1/AI koeff"=w196) -> ("P0"=w233:dbl[], "P1"=w234:dbl[], "P2"=w235:dbl[])
      n153 = Close File(refnum=w218, error in=w217) -> (path=w212:path)  [unwired: 1 out]
      "schnelle Heizungen" <- string[] ["Trap1 [°C]", "Trap2 [°C]", "PreCol1 [°C]", "PreCol2 [°C]", "MainCol1 [°C]", "MainCol2 [°C]"]
    }
    frame #1 {
      w303 = dbl[] [-1.0]
      w366 = 0
      w343 = 0 ("Zyklusnummer1")
      n154 = Add Array Elements(numeric array=w319) -> (sum=w318:i32)
      n155 = Array Size(array=w327) -> (size(s)=w346:i32)
      n156 = Unbundle(w342) -> ("created path"=w341:path, "created path"=w339:path, "created path"=w338:path, "Dateiname Housekeeping"=w340:string, "DateinameECD1"=w337:string, "DateinameECD2"=w336:string, "tdms0"=w335:refnum<k34>, "tdms1"=w334:refnum<k34>, "tdms0"=w333:refnum<k34>, "tdms1"=w332:refnum<k34>, "tdms0"=w331:refnum<k34>, "tdms1"=w330:refnum<k34>)
      n157 = Index Array(array=w320, index #1=0 ("Index"), index #2=1 ("Index"), index #3=2 ("Index"), index #4=3 ("Index")) -> (element #1=w355:i32, element #2=w354:i32, element #3=w357:i32, element #4=w356:i32)
      n158 = while {
        shift-right: ["Methode"] -> _
        shift-left: w392 -> [w1037]
        stop <- w1039 stop-if-true
        n159 = call "Bis zum nächsten Vielfachen warten7"("Count(mSec)"=u32 1000) -> ()  [unwired: 1 out]
        n160 = Not Equal?(x=w1037, y="Methode") -> (x != y?=w1035:bool)
        n161 = global read "gvbooleschRT.vi" "global stop RT"() -> (w1039:bool)
        n162 = global write "GVMethodenwechsel.vi" "Methodenwechsel?"(w1035) -> ()
      }
      n163 = call <vilib>:"Space Constant.vi"() -> ("String"=w305:string)
      n164 = while {
        tunnel: w323 -> [w549]
        tunnel: w388 -> [w552]
        tunnel: w387 -> [w551]
        tunnel: w386 -> [w550]
        shift-right: [w554] -> _
        shift-left: errorcluster {"status"=FALSE, "code"=0, "source"=""} ("error out") -> [w553]
        stop <- w555 stop-if-true
        n165 = call "AIsFIFORT_ECD.vi"("FPGA-VI-Referenz"=w549, "P2"=w552, "P1"=w551, "P0"=w550, "error in"=w553) -> ("error out"=w554:errorcluster)
        "AIsFIFOread" <- w554
        n166 = global read "gvbooleschRT.vi" "global stop RT"() -> (w555:bool)
      }
      n167 = while {
        tunnel: w323 -> [w556]
        tunnel: w302 -> [w559]
        tunnel: w301 -> [w558]
        tunnel: w300 -> [w557]
        shift-right: [w561] -> _
        shift-left: errorcluster {"status"=FALSE, "code"=0, "source"=""} ("error out") -> [w560]
        stop <- w563 stop-if-true
        n168 = call "Bis zum nächsten Vielfachen warten16"("Count(mSec)"=u32 100) -> ()  [unwired: 1 out]
        n169 = call "TrapsMachMitteln_ECD.vi"("FPGA-VI-Referenz"=w556, "Traps/MachKoeff2"=w559, "Traps/MachKoeff1"=w558, "Traps/MachKoeff0"=w557, "error in"=w560) -> ("error out"=w561:errorcluster)
        "MWTrapsMachs" <- w561
        n170 = global read "gvbooleschRT.vi" "global stop RT"() -> (w563:bool)
      }
      n171 = for {
        N: 1 -> [_]
        tunnel: w323 -> [w564]
        tunnel: [w564] -> w348
        n172 = call "Warten8"("Count(mSec)"=u32 100) -> ()  [unwired: 1 out]
      }
      n173 = Build Array(w305) -> (w304:string[])
      n174 = Initialize Array(-1 ("Element"), 4 ("Dimension")) -> (w321:i32[])
      n175 = global read "GVVentilposition.vi" "Ventilposition"() -> (w329:i32)
      n176 = Add(x=w357, y=w356) -> (x+y=w353:i32)
      n177 = Bundle(w304, w304, w304) -> (w364:cluster{string[], string[], string[]})  [unwired: 1 in]
      n178 = Index Array(array=w314, index=w312) -> (element=w313:T7)
      n179 = Initialize Array(cluster{"output high":dbl, "output low":dbl} {"output high"=99999.0, "output low"=0.0} ("output range"), w346) -> (w328:cluster{"output high":dbl, "output low":dbl}[])
      n180 = Build Array(w355, w354, w353) -> (w293:i32[])
      n181 = case shown="True" TRUE ("HKSpeichern") {
        tunnel: w390 -> [_ w542]
        frame False {
        }
        frame True {
          n182 = while {
            tunnel: w542 -> [w546]
            shift-right: [w544] -> _
            shift-left: errorcluster {"status"=FALSE, "code"=0, "source"=""} ("error out") -> [w543]
            stop <- w548 stop-if-true
            n183 = call "Bis zum nächsten Vielfachen warten2"("Count(mSec)"=u32 1000) -> ()  [unwired: 1 out]
            n184 = local read "Methode"() -> (w545:i32)
            n185 = global read "gvbooleschRT.vi" "global stop RT"() -> (w548:bool)
            n186 = call "HKinTDMS-01-16.vi"("Methode"=w545, "error in (no error)"=w543, "Kanäle"=w546) -> ("error out"=w544:errorcluster)
            "TDMSwriteHK" <- w544
          }
        }
      }
      n187 = while {
        tunnel: w391 -> [w678]
        shift-right: [w677] -> _
        shift-left: w314 -> [w659]
        tunnel: w328 -> [w676]
        tunnel: w327 -> [w675]
        tunnel: w323 -> [w674]
        tunnel: w326 -> [w673]
        tunnel: w325 -> [w672]
        shift-right: [w666] -> _
        shift-left: 0 -> [w671]
        tunnel: w323 -> [w670]
        tunnel: w322 -> [w669]
        shift-right: [w665] -> _
        shift-left: w321 -> [w668]
        tunnel: w320 -> [w660]
        tunnel: w319 -> [w661]
        tunnel: w318 -> [w662]
        tunnel: w317 -> [w663]
        tunnel: w316 -> [w664]
        tunnel: w315 -> [w667]
        shift-right: [w583] -> _
        shift-left: w313 -> [w582]
        tunnel: w302 -> [w568]
        tunnel: w301 -> [w569]
        tunnel: w300 -> [w570]
        tunnel: w295 -> [w571]
        tunnel: w291 -> [w566]
        i -> [w586]
        stop <- w679 stop-if-true
        w576 = 0  # ZeileMainMach2
        w577 = 0  # ZeileMainMach1
        w627 = FALSE
        w626 = 0.0
        w628 = 0  # ZeilennummerMPV
        w632 = cluster{dbl[], dbl[]} {[], []}
        w641 = dbl[] []
        w645 = 0  # ZeilePreMach2
        w646 = 0  # ZeilePreMach1
        w647 = 0  # ZeileFPGAFixp
        w648 = 0  # ZeileFPGAPID
        w649 = 0  # ZeileFPGABoolesch
        w650 = i32[] [0, 0, 0, 0]  # ZeilennummernHorst
        w651 = i32[] [0, 0, 0, 0]  # ZeilennummernDIOs
        n188 = Unbundle(w582) -> ("Zykluslängen [s]"=w567:dbl[], "ZeitpktDIOsMod0"=w625:dbl[], "ZeitpktDIOsMod1"=w624:dbl[], "ZeitpktDIOsMod2A"=w623:dbl[], "ZeitpktDIOsMod2B"=w622:dbl[], "DIOsSPMod0"=w621:bool[][], "DIOsSPMod1"=w620:bool[][], "DIOsSPMod2A"=w619:bool[][], "DIOsSPMod2B"=w618:bool[][], "Mod0HorstZeitpkt"=w617:dbl[], "Mod1HorstZeitpkt"=w616:dbl[], "Mod2AHorstZeitpkt"=w615:dbl[], "Mod2BHorstZeitpkt"=w614:dbl[], "HorstSPMod0"=w613:dbl[][], "HorstSPMod1"=w612:dbl[][], "HorstSPMod2A"=w611:dbl[][], "HorstSPMod2B"=w610:dbl[][], "LHSetpoints"=w609:dbl[], "LHHeizen?"=w608:bool[], "ZPktFPGABoolesch"=w607:dbl[], "FPGABoolesch"=w606:bool[][], "ZeitpktFPGAPID"=w605:dbl[], "FPGAPID"=w604:T10, "ZeitpktFPGAFixp"=w603:dbl[], w602:dbl[][], "t_PreMach1"=w601:dbl[], "T_PreMach1"=w600:dbl[], "t_PreMach2"=w599:dbl[], "T_PreMach2"=w598:dbl[], "PIDs für \"träge\" Heizungen"=w597:T11, "Zwangsbedingungen"=w596:dbl[][], "Dateien fürs MS schicken?"=w595:bool, "ZeitpunkteMPV"=w594:dbl[], "SPMPV"=w593:i32[], "ZeitpktMS-1"=w592:dbl, "ZeitpktMS-2"=w591:dbl, "Int.Start1"=w590:dbl, "Int.Stop1"=w589:dbl, "Int.Start2"=w588:dbl, "Int.Stop2"=w587:dbl, "t_MainMach1"=w581:dbl[], "T_MainMach1"=w580:dbl[], "t_MainMach2"=w579:dbl[], "T_MainMach2"=w578:dbl[])  [unwired: 1 out]
        n189 = while {
          tunnel: w567 -> [w696]
          tunnel: w566 -> [w688]
          stop <- w681 stop-if-true
          n190 = global read "GVZeitenZyklen.vi" "Big Ben, Methodenzeit, Zykluszeit0, Zykluszeit1, Zykluszeit2A, Zykluszeit2B"() -> (w699:dbl[])
          n191 = call "Bis zum nächsten Vielfachen warten19"("Count(mSec)"=u32 500) -> ()  [unwired: 1 out]
          n192 = global read "GVZeitenZyklen.vi" "ZyklusNummernGesamt"() -> (w686:i32[])
          n193 = Index Array(array=w696, index=2 ("Index")) -> (element=w692:dbl)
          n194 = Subtract(x=w692, y=1.0) -> (x-y=w690:dbl)
          n195 = Index Array(array=w699, index=4 ("Index")) -> (element=w697:dbl)
          n196 = global read "GVChroms.vi" "ECD1Chrom"() -> (w693:dbl[])
          n197 = Greater Or Equal?(x=w697, y=w690) -> (x >= y?=w694:bool)
          n198 = Index Array(array=w686, index=2 ("Index")) -> (element=w685:i32)
          n199 = case shown="True" w694 {
            tunnel: w693 -> [_ w702]
            tunnel: w688 -> [_ w701]
            tunnel: w685 -> [_ w700]
            frame False {
            }
            frame True {
              n200 = flat-sequence {
                tunnel: w702 -> [w713]
                tunnel: w701 -> [w709]
                tunnel: w700 -> [w708]
                frame #0 {
                  n201 = Number To Decimal String(number=w708, width (-)=i16 4 ("Breite (-)")) -> (decimal integer string=w706:string)
                  n202 = Concatenate Strings(w706, ".hag" ("String")) -> (w704:string)
                  n203 = Build Path(base path=w709, name or relative path=w704) -> (appended path=w703:path)
                  n204 = Open/Create/Replace File(file path (use dialog)=w703, operation (0:open)=T4."replace or create" ("Operation (0:Öffnen)")) -> (refnum out=w715:refnum<file>, error out=w714:errorcluster)  [unwired: 4 in, 1 out]
                  n205 = Write to Binary File(file (use dialog)=w715, data=w713, error in=w714) -> (refnum out=w712:refnum<file>, error out=w711:errorcluster)  [unwired: 3 in, 1 out]
                  n206 = Close File(refnum=w712, error in=w711) -> (error out=→"Fehler ECD1alt":errorcluster)  [unwired: 1 out]
                }
                frame #1 {
                  n207 = call "Warten3"("Count(mSec)"=u32 2000) -> ()  [unwired: 1 out]
                }
              }
            }
          }
          n208 = global read "GVMethodenwechsel.vi" "Methodenwechsel?"() -> (w682:bool)
          n209 = global read "gvbooleschRT.vi" "global stop RT"() -> (w683:bool)
          n210 = Or(x=w682, y=w683) -> (x .or. y?=w684:bool)
          n211 = local read "veränderte Methode benutzen"() -> (w680:bool)
          n212 = Or(x=w684, y=w680) -> (x .or. y?=w681:bool)
        }
        n213 = Add(x=w668, y=1) -> (x+y=w636:i32[])
        n214 = local read "Methode"() -> (w585:i32)
        n215 = Build Cluster Array(w621, w620, w619, w618) -> (w655:cluster{"DIOsSPMod2B":bool[][]}[])
        n216 = Build Cluster Array(w613, w612, w611, w610) -> (w653:cluster{"HorstSPMod2B":dbl[][]}[])
        n217 = Build Cluster Array(w625, w624, w623, w622) -> (w656:cluster{"ZeitpktDIOsMod2B":dbl[]}[])
        n218 = Build Cluster Array(w617, w616, w615, w614) -> (w654:cluster{"Mod2BHorstZeitpkt":dbl[]}[])
        n219 = while {
          tunnel: w661 -> [w786]
          tunnel: w664 -> [w779]
          tunnel: w663 -> [w780]
          tunnel: w660 -> [w785]
          tunnel: w662 -> [w781]
          tunnel: w596 -> [w782]
          stop <- w788 stop-if-true
          n220 = call "Bis zum nächsten Vielfachen warten10"("Count(mSec)"=u32 1000) -> ()  [unwired: 1 out]
          n221 = local read "Methode"() -> (w784:i32)
          n222 = global read "GVMethodenwechsel.vi" "Methodenwechsel?"() -> (w790:bool)
          n223 = global read "gvbooleschRT.vi" "global stop RT"() -> (w791:bool)
          n224 = case shown="True" "global stop RT" {
            frame False {
            }
            frame True {
              n225 = global write "gvbooleschRT.vi" "global stop RT"(TRUE ("global stop RT")) -> ()
            }
          }
          n226 = call "ZwangsbedingungenGV-15-07-17.vi"("AnzahlHorst"=w779, "AnzahlHorst/Modul"=w785, "AnzahlLH"=w780, "AnzahlDIOs/Modul"=w786, "AnzahlDIOs"=w781, "Zwangsbedingungen"=w782, "Methodennummer"=w784) -> ("Methodennummer"=w783:i32)  [unwired: 4 in]
          n227 = local write "Methode"(w783) -> ()
          n228 = local read "veränderte Methode benutzen"() -> (w789:bool)
          n229 = Compound Arithmetic op=OR(w791, w790, w789) -> (w788:bool)
        }
        n230 = Equal?(x=w586, y=0) -> (x = y?=w657:bool)
        n231 = global read "GVZeitenZyklen.vi" "ZyklusNummern"() -> (w635:i32[])
        n232 = global read "GVZwangs.vi" "ZwangsHorst?"() -> (w640:cluster{bool[]}[])
        n233 = global read "gvbooleschRT.vi" "global stop RT"() -> (w679:bool)
        n234 = global read "GVZwangsMPV.vi" "ZwangsMPV?"() -> (w574:bool)
        n235 = global read "GVZwangs.vi" "ZwangsDIO?"() -> (w639:cluster{bool[]}[])
        n236 = global read "GVaktuelleTDMS.vi" "aktuelleTDMS-DateiECD1"() -> (w634:refnum<k34>)
        n237 = while {
          tunnel: w675 -> [w769]
          tunnel: w676 -> [w772]
          tunnel: w674 -> [w773]
          tunnel: w609 -> [w770]
          tunnel: w597 -> [w771]
          shift-right: [w767] -> _
          shift-left: errorcluster {"status"=FALSE, "code"=0, "source"=""} ("error out") -> [w768]
          stop <- w774 stop-if-true
          n238 = call "LH_ECD.vi"("FPGA-VI-Referenz"=w773, "OutputRange"=w772, "LHSetpoints"=w770, "AIsLH"=w769, "error in"=w768, "LH-Gruppe"="LH-Gruppe", "PIDs für \"träge\" Heizungen"=w771) -> ("error out"=w767:errorcluster)
          "LH" <- w767
          n239 = call "Bis zum nächsten Vielfachen warten12"("Count(mSec)"=u32 100) -> ()  [unwired: 1 out]
          n240 = global read "GVMethodenwechsel.vi" "Methodenwechsel?"() -> (w776:bool)
          n241 = global read "gvbooleschRT.vi" "global stop RT"() -> (w777:bool)
          n242 = local read "veränderte Methode benutzen"() -> (w775:bool)
          n243 = Compound Arithmetic op=OR(w777, w776, w775) -> (w774:bool)
        }
        n244 = while {
          shift-right: [w730] -> _
          shift-left: w627 -> [w734]
          shift-right: [w729] -> _
          shift-left: w626 -> [w733]
          shift-right: [w728] -> _
          shift-left: w627 -> [w732]
          shift-right: [w727] -> _
          shift-left: w626 -> [w731]
          tunnel: w667 -> [w726]
          tunnel: w590 -> [w721]
          tunnel: w589 -> [w720]
          tunnel: w588 -> [w719]
          tunnel: w587 -> [w718]
          stop <- w723 stop-if-true
          n245 = call "Integrieren.vi"("Integrieren1"=w734, "Integral1"=w733, "Integrieren2"=w732, "Integral2"=w731, "Int.Start1"=w721, "Int.Stop1"=w720, "Int.Start2"=w719, "HorstProbenflußNr."=w726, "Int.Stop2"=w718) -> ("Integrieren1"=w730:bool, "Integral1"=w729:dbl, "Integrieren2"=w728:bool, "Integral2"=w727:dbl)  [unwired: 7 in]
          n246 = call "Bis zum nächsten Vielfachen warten9"("Count(mSec)"=u32 100) -> ()  [unwired: 1 out]
          n247 = global read "GVMethodenwechsel.vi" "Methodenwechsel?"() -> (w724:bool)
          n248 = global read "gvbooleschRT.vi" "global stop RT"() -> (w725:bool)
          n249 = local read "veränderte Methode benutzen"() -> (w722:bool)
          n250 = Compound Arithmetic op=OR(w725, w724, w722) -> (w723:bool)
        }
        n251 = while "Zeit" {
          tunnel: w657 -> [w974]
          tunnel: w567 -> [w972]
          tunnel: w636 -> [w967]
          tunnel: [w966] -> w665
          shift-right: [w963] -> _
          shift-left: 0.0 -> [w964]
          i -> [w976]
          stop <- w969 stop-if-true
          n252 = Equal?(x=w976, y=0) -> (x = y?=w965:bool)
          n253 = call "Bis zum nächsten Vielfachen warten15"("Count(mSec)"=u32 50) -> ()  [unwired: 1 out]
          n254 = call "BigBen_ECD.vi"("MethodenStartzeit"=w964, "Methodenstart?"=w965, "Programmstart?"=w974, "Zykluslängen [s]"=w972, "MethodenStartZyklusNummern"=w967) -> ("MethodenStartzeit"=w963:dbl, "ZyklusNummernGesamt"=w966:i32[])  [unwired: 2 in]
          n255 = global read "GVMethodenwechsel.vi" "Methodenwechsel?"() -> (w968:bool)
          n256 = global read "gvbooleschRT.vi" "global stop RT"() -> (w973:bool)
          n257 = Or(x=w968, y=w973) -> (x .or. y?=w970:bool)
          n258 = local read "veränderte Methode benutzen"() -> (w971:bool)
          n259 = Or(x=w971, y=w970) -> (x .or. y?=w969:bool)
        }
        n260 = Bundle(w656, w655, w654, w653, "LHHeizen?"=w608, "ZPktFPGABoolesch"=w607, "FPGABoolesch"=w606, "ZeitpktFPGAPID"=w605, "FPGAPID"=w604, "ZeitpktFPGAFixp"=w603, w602, "t_PreMach1"=w601, "T_PreMach1"=w600, "t_PreMach2"=w599, "T_PreMach2"=w598, "ZeitpunkteMPV"=w594, "SPMPV"=w593, "t_MainMach1"=w581, "T_MainMach1"=w580, "t_MainMach2"=w579, "T_MainMach2"=w578) -> (w652:T12)  [unwired: 1 in]
        n261 = Index Array(array=w659, index=w585) -> (element=w584:T7)
        n262 = global read "GVZwangs.vi" "ZwangsFPGABoolesch?"() -> (w638:bool[])
        n263 = while {
          tunnel: w678 -> [w989]
          shift-right: [w980] -> _
          shift-left: w584 -> [w988]
          tunnel: w585 -> [w986]
          shift-right: [w978] -> w677
          shift-left: w659 -> [w987]
          tunnel: [w979] -> w583
          stop <- w982 stop-if-true
          n264 = call "Bis zum nächsten Vielfachen warten8"("Count(mSec)"=u32 500) -> ()  [unwired: 1 out]
          n265 = global read "GVMethodenwechsel.vi" "Methodenwechsel?"() -> (w984:bool)
          n266 = global read "gvbooleschRT.vi" "global stop RT"() -> (w983:bool)
          n267 = case shown="True" "Methode verändern" {
            tunnel: w989 -> [_ w1011]
            tunnel: w988 -> [w1008 w1010]
            tunnel: [w1008 w1009] -> w980
            frame False {
            }
            frame True {
              n268 = call "methodeändern-15-07-17.vi"("->Methode"=w1010, "Namen"=w1011) -> ("Methode->"=w1009:T13)  [unwired: 1 in]
              n269 = property on="Methode verändern" class="Bool. (strikt)"("Value"=FALSE ("Methode verändern")) -> ()  [unwired: 2 in, 2 out]
            }
          }
          n270 = Compound Arithmetic op=OR(w984, w983, "veränderte Methode benutzen") -> (w982:bool)
          n271 = case shown="True" "Methode speichern" {
            tunnel: w980 -> [_ w1005]
            tunnel: w987 -> [w998 w1007]
            tunnel: w986 -> [_ w1006]
            tunnel: [w998 w1000] -> w978
            frame False {
            }
            frame True {
              n272 = Replace Array Subset(array=w1007, new element=w1005, index=w1006) -> (w1000:T3)
              n273 = property on="Methode speichern" class="Bool. (strikt)"("Value"=FALSE ("Methode speichern")) -> ()  [unwired: 2 in, 2 out]
              n274 = Open/Create/Replace File(file path (use dialog)=path "c:/methoden.pery" ("Dateipfad (Dialog verwenden)"), operation (0:open)=T4."replace" ("Operation (0:Öffnen)")) -> (refnum out=w1002:refnum<file>)  [unwired: 4 in, 2 out]
              n275 = Write to Binary File(file (use dialog)=w1002, data=w1000) -> (refnum out=w999:refnum<file>)  [unwired: 4 in, 2 out]
              n276 = Close File(refnum=w999) -> ()  [unwired: 1 in, 2 out]
            }
          }
          n277 = case shown="False" "veränderte Methode benutzen" {
            tunnel: w980 -> [_ w995]
            tunnel: [w992 w995] -> w979
            tunnel: w978 -> [w994 _]
            frame False {
              n278 = local read "Methode"() -> (w993:i32)
              n279 = Index Array(array=w994, index=w993) -> (element=w992:T7)
            }
            frame True {
              n280 = flat-sequence {
                frame #0 {
                  n281 = call "Warten"("Count(mSec)"=u32 1100) -> ()  [unwired: 1 out]
                }
                frame #1 {
                  n282 = property on="veränderte Methode benutzen" class="Bool. (strikt)"("Value"=FALSE ("Methode verändern")) -> ()  [unwired: 2 in, 2 out]
                }
              }
            }
          }
        }
        n283 = Bundle(w641, w641, w641, w641) -> (w642:cluster{dbl[], dbl[], dbl[], dbl[]})  [unwired: 1 in]
        n284 = Bundle("ZyklusNummern"=w635, "ZeilennummernDIOs"=w651, "ZwangsDIO?"=w639, "ZeilennummernHorst"=w650, "ZwangsHorst?"=w640, "ZeileFPGABoolesch"=w649, "ZwangsFPGABoolesch?"=w638, "ZeileFPGAPID"=w648, "ZeileFPGAFixp"=w647, "ZeilePreMach1"=w646, "ZeilePreMach2"=w645, "ZeilennummerMPV"=w628, "ZeileMainMach1"=w577, "ZeileMainMach2"=w576, "ZwangsMPV?"=w574) -> (w644:T14)  [unwired: 1 in]
        n285 = while {
          shift-right: [w906] -> _
          shift-left: w642 -> [w913]
          shift-right: [w905] -> _
          shift-left: w642 -> [w912]
          shift-right: [w903] -> _
          shift-left: T5 {"Zyklus1"=0, "Zeitachse1"=0, "dargestellte Größe 1"=0, "Zyklus2"=0, "Zeitachse2"=0, "dargestellte Größe 2"=0} ("AnzeigeEinstellungen") -> [w911]
          tunnel: w567 -> [w881]
          shift-right: [w877] -> _
          shift-left: w634 -> [w876]
          shift-right: [w872] -> _
          shift-left: w632 -> [w874]
          shift-right: [w861] -> _
          shift-left: w632 -> [w873]
          shift-right: ["Detektor"] -> _
          shift-left: 0 ("Detektor") -> [w870]
          tunnel: w571 -> [w859]
          stop <- w917 stop-if-true
          w882 = 0.0 ("X-Achse.Bereich:Minimum")
          n286 = Unbundle(w859) -> ("Modul1/AI sicherer Bereich"=w852:dbl[][], "Modul2/AI sicherer Bereich"=w837:dbl[][], "Modul3/AI sicherer Bereich"=w828:dbl[][], "Traps/Machs sicherer Bereich"=w819:dbl[][], w811:dbl[][], "Metavariablen grüner Bereich"=w802:dbl[][])
          n287 = call "Bis zum nächsten Vielfachen warten14"("Count(mSec)"=u32 1000) -> ()  [unwired: 1 out]
          n288 = global read "GVMWHorst.vi" "MWHorst"() -> (w810:dbl[])
          "MWHorst" <- w810
          n289 = case shown="0, Standard" "Detektor" {
            tunnel: [w927 w939] -> w872
            tunnel: w881 -> [w926 w941]
            tunnel: "Detektor" -> [w921 w935]
            tunnel: [w925 w940] -> w879
            tunnel: [w924 w938] -> w877
            frame 0, Default {
              n290 = Increment(x=w921) -> (x+1=w922:i32)
              n291 = Increment(x=w922) -> (x+1=w920:i32)
              n292 = global read "GVChroms.vi" "ECD1Chrom"() -> (w923:dbl[])
              n293 = global read "GVaktuelleTDMS.vi" "aktuelleTDMS-DateiECD1"() -> (w924:refnum<k34>)
              n294 = Index Array(array=w926, index=w920) -> (element=w925:dbl)
              n295 = Array Size(array=w923) -> (size(s)=w929:i32)
              n296 = for {
                N: w929 -> [_]
                tunnel: [w930] -> w928 mode=indexing
                i -> [w933]
                n297 = To Double Precision Float(number=w933) -> (double precision float=w932:dbl)
                n298 = Divide(x=w932, y=10.0) -> (x/y=w930:dbl)
              }
              n299 = Bundle(w928, "ECD1Chrom"=w923) -> (w927:cluster{dbl[], "ECD1Chrom":dbl[]})  [unwired: 1 in]
            }
            frame 1 {
              n300 = Increment(x=w935) -> (x+1=w936:i32)
              n301 = Increment(x=w936) -> (x+1=w934:i32)
              n302 = global read "GVChroms.vi" "ECD2Chrom"() -> (w937:dbl[])
              n303 = global read "GVaktuelleTDMS.vi" "aktuelleTDMS-DateiECD2"() -> (w938:refnum<k34>)
              n304 = Index Array(array=w941, index=w934) -> (element=w940:dbl)
              n305 = Array Size(array=w937) -> (size(s)=w943:i32)
              n306 = for {
                N: w943 -> [_]
                tunnel: [w944] -> w942 mode=indexing
                i -> [w947]
                n307 = To Double Precision Float(number=w947) -> (double precision float=w946:dbl)
                n308 = Divide(x=w946, y=10.0) -> (x/y=w944:dbl)
              }
              n309 = Bundle(w942, "ECD2Chrom"=w937) -> (w939:cluster{dbl[], "ECD2Chrom":dbl[]})  [unwired: 1 in]
            }
          }
          n310 = Subtract(x="DetYMax", y="DetYMin") -> (x-y=w887:dbl)
          n311 = Subtract(x="HK1YMax", y="HK1YMin") -> (x-y=w897:dbl)
          n312 = Subtract(x="HK2YMax", y="HK2YMin") -> (x-y=w892:dbl)
          n313 = Equal?(x="Detektor", y=w870) -> (x = y?=w869:bool)
          n314 = Index Array(array=w852, index (col) #1=0 ("disabled index (col)"), index (col) #2=1 ("index (col)")) -> (element #1=w849:dbl[], element #2=w847:dbl[])  [unwired: 2 in]
          n315 = Index Array(array=w837, index (col) #1=0 ("disabled index (col)"), index (col) #2=1 ("index (col)")) -> (element #1=w841:dbl[], element #2=w840:dbl[])  [unwired: 2 in]
          n316 = Index Array(array=w819, index (col) #1=0 ("disabled index (col)"), index (col) #2=1 ("index (col)")) -> (element #1=w823:dbl[], element #2=w822:dbl[])  [unwired: 2 in]
          n317 = Index Array(array=w811, index (col) #1=0 ("disabled index (col)"), index (col) #2=1 ("index (col)")) -> (element #1=w815:dbl[], element #2=w814:dbl[])  [unwired: 2 in]
          n318 = Index Array(array=w828, index (col) #1=0 ("disabled index (col)"), index (col) #2=1 ("index (col)")) -> (element #1=w832:dbl[], element #2=w831:dbl[])  [unwired: 2 in]
          n319 = Index Array(array=w802, index (col) #1=0 ("disabled index (col)"), index (col) #2=1 ("index (col)")) -> (element #1=w806:dbl[], element #2=w805:dbl[])  [unwired: 2 in]
          n320 = global read "GVMethodenwechsel.vi" "Methodenwechsel?"() -> (w915:bool)
          n321 = global read "GVZeitenZyklen.vi" "ZyklusNummern"() -> (w884:i32[])
          "ZyklusNummern" <- w884
          n322 = global read "gvbooleschRT.vi" "global stop RT"() -> (w916:bool)
          n323 = global read "GVMetavariablen.vi" "Metavariablen"() -> (w801:dbl[])
          "Metavariablen" <- w801
          n324 = global read "GVVentilposition.vi" "Ventilposition"() -> (→"Ventilposition":i32)
          n325 = global read "GVZeitenZyklen.vi" "ZyklusNummernGesamt"() -> (→"ZyklusNummernGesamt":i32[])
          n326 = Divide(x=w887, y=20.0) -> (x/y=w885:dbl)
          n327 = Divide(x=w897, y=10.0) -> (x/y=w895:dbl)
          n328 = Divide(x=w892, y=10.0) -> (x/y=w890:dbl)
          n329 = local read "veränderte Methode benutzen"() -> (w914:bool)
          n330 = Or(x=w915, y=w916) -> (x .or. y?=w918:bool)
          n331 = Greater Or Equal?(x=w810, y=w815) -> (x >= y?=w813:bool[])
          n332 = Less Or Equal?(x=w810, y=w814) -> (x <= y?=w812:bool[])
          n333 = Greater Or Equal?(x=w801, y=w806) -> (x >= y?=w804:bool[])
          n334 = Less Or Equal?(x=w801, y=w805) -> (x <= y?=w803:bool[])
          n335 = global read "GVHK1Hz.vi" "Mod1Mod2Mod3/AITrapsMachs1Hz"() -> (w797:dbl[])
          n336 = And(x=w813, y=w812) -> (x .and. y?=→"HorstOK?":bool[])
          n337 = And(x=w804, y=w803) -> (x .and. y?=→"MVOK?":bool[])
          n338 = Or(x=w918, y=w914) -> (x .or. y?=w917:bool)
          n339 = global write "GVMetavariablen.vi" "MV-Festhalten"("MV-Festhalten") -> ()
          n340 = global read "GVZeitenZyklen.vi" "Big Ben, Methodenzeit, Zykluszeit0, Zykluszeit1, Zykluszeit2A, Zykluszeit2B"() -> (w864:dbl[])
          n341 = global write "GVMetavariablen.vi" "MV-Vorgaben"("MV-Vorgaben") -> ()
          n342 = Array Subset(array=w797, index=0 ("Index"), length=32 ("Länge")) -> (w848:dbl[])
          "AIs1" <- w848
          n343 = Array Subset(array=w797, index=32 ("Index"), length=32 ("Länge")) -> (w836:dbl[])
          "AIs2" <- w836
          n344 = Array Subset(array=w797, index=96 ("Index"), length=6 ("Länge")) -> (w796:dbl[])
          "schnelle Heizungen" <- w796
          n345 = Array Subset(array=w797, index=64 ("Index"), length=32 ("Länge")) -> (w827:dbl[])
          "AIs3" <- w827
          n346 = Greater Or Equal?(x=w796, y=w823) -> (x >= y?=w821:bool[])
          n347 = Less Or Equal?(x=w796, y=w822) -> (x <= y?=w820:bool[])
          n348 = Greater Or Equal?(x=w848, y=w849) -> (x >= y?=w846:bool[])
          n349 = Less Or Equal?(x=w848, y=w847) -> (x <= y?=w845:bool[])
          n350 = Greater Or Equal?(x=w836, y=w841) -> (x >= y?=w839:bool[])
          n351 = Less Or Equal?(x=w836, y=w840) -> (x <= y?=w838:bool[])
          n352 = And(x=w821, y=w820) -> (x .and. y?=→"SHOK?":bool[])
          n353 = Greater Or Equal?(x=w827, y=w832) -> (x >= y?=w830:bool[])
          n354 = Less Or Equal?(x=w827, y=w831) -> (x <= y?=w829:bool[])
          n355 = And(x=w846, y=w845) -> (x .and. y?=→"AIs1OK?":bool[])
          n356 = And(x=w839, y=w838) -> (x .and. y?=→"AIs2OK?":bool[])
          n357 = And(x=w830, y=w829) -> (x .and. y?=→"AIs3OK?":bool[])
          n358 = To Long Integer(number=w864) -> (32bit integer=→"Big Ben, Methodenzeit, Zykluszeit0, Zykluszeit1, Zykluszeit2A, Zykluszeit2B":i32[])
          n359 = Equal?(x=w877, y=w876) -> (x = y?=w875:bool)
          n360 = call "AnzeigeGV.vi"("veränderte Methode benutzen"=w914, "Zykluslängen [s]"=w881, "Cluster1"=w913, "Big Ben, Methodenzeit, Zykluszeit0, Zykluszeit1, Zykluszeit2A, Zykluszeit2B"=w864, "Zyklusnummern 0, 1, 2A, 2B"=w884, "Cluster2"=w912, "AnzeigeEinstellungen"=w911, "dargestellte Größe 1"="dargestellte Größe 1", "Zeitachse1"="Zeitachse1", "dargestellte Größe 2"="dargestellte Größe 2", "Zeitachse2"="Zeitachse2") -> ("Anzeige2"=→"Housekeeping2":cluster{dbl[], dbl[]}, "Cluster1"=w906:cluster{dbl[], dbl[], dbl[], dbl[]}, "x1Inkr"=w901:dbl, "Cluster2"=w905:cluster{dbl[], dbl[], dbl[], dbl[]}, "Anzeige1"=→"Housekeeping1":cluster{dbl[], dbl[]}, "AnzeigeEinstellungen"=w903:T5, "x2Max"=w865:dbl, "x2Inkr"=w900:dbl, "x1Max"=w866:dbl)  [unwired: 8 in]
          n361 = Divide(x=w879, y=20.0) -> (x/y=w880:dbl)
          n362 = property on="Detektor 2" class="XYGraph (strikt)"("XScale.Minimum"=w882, "XScale.Maximum"=w879, "XScale.Increment"=w880, "YScale.Minimum"="DetYMin", "YScale.Maximum"="DetYMax", "YScale.Increment"=w885) -> ()  [unwired: 2 in, 2 out]
          n363 = property on="Housekeeping1" class="XYGraph (strikt)"("XScale.Minimum"=w882, "XScale.Maximum"=w866, "XScale.Increment"=w901, "YScale.Minimum"="HK1YMin", "YScale.Maximum"="HK1YMax", "YScale.Increment"=w895) -> ()  [unwired: 2 in, 2 out]
          n364 = property on="Housekeeping2" class="XYGraph (strikt)"("XScale.Minimum"=w882, "XScale.Maximum"=w865, "XScale.Increment"=w900, "YScale.Minimum"="HK2YMin", "YScale.Maximum"="HK2YMax", "YScale.Increment"=w890) -> ()  [unwired: 2 in, 2 out]
          n365 = Select(t=w873, s=w875, f=w874) -> (s? t:f=w868:cluster{dbl[], dbl[]})
          n366 = Select(t=w868, s=w869, f=cluster{dbl[], dbl[]} {[], []} ("s? t:f")) -> (s? t:f=w861:cluster{dbl[], dbl[]})
          n367 = Build Array(w872, w861) -> (→"Detektor 2":cluster{dbl[], "ECD2Chrom":dbl[]}[])
        }
        n368 = while "ZyklusSteuerung" {
          tunnel: w669 -> [w952]
          tunnel: w670 -> [w948]
          shift-right: [w950] -> _
          shift-left: w644 -> [w956]
          tunnel: w652 -> [w957]
          tunnel: w570 -> [w953]
          tunnel: w569 -> [w954]
          tunnel: w568 -> [w955]
          shift-right: [w949] -> _
          shift-left: errorcluster {"status"=FALSE, "code"=0, "source"=""} ("error out") -> [w951]
          stop <- w958 stop-if-true
          n369 = call "Bis zum nächsten Vielfachen warten11"("Count(mSec)"=u32 100) -> ()  [unwired: 1 out]
          n370 = global read "GVMethodenwechsel.vi" "Methodenwechsel?"() -> (w961:bool)
          n371 = global read "gvbooleschRT.vi" "global stop RT"() -> (w960:bool)
          n372 = local read "veränderte Methode benutzen"() -> (w959:bool)
          n373 = Compound Arithmetic op=OR(w961, w960, w959) -> (w958:bool)
          n374 = call "ZyklussteuerungGV_ECD.vi"("Traps/MachKoeff0"=w953, "DIOsNummern"=w952, "error in"=w951, "Traps/MachKoeff1"=w954, "FPGA-VI-Referenz"=w948, "Traps/MachKoeff2"=w955, "Schieberegister"=w956, "Zeitpunkte/Setpoints"=w957) -> ("Schieberegister"=w950:T15, "error out"=w949:errorcluster)  [unwired: 6 in]
          "Zyklus" <- w949
        }
        n375 = global read "GVZeitenZyklen.vi" "Big Ben, Methodenzeit, Zykluszeit0, Zykluszeit1, Zykluszeit2A, Zykluszeit2B"() -> (w631:dbl[])
        n376 = Index Array(array=w631, index=3 ("Index")) -> (element=w629:dbl)
        n377 = while {
          tunnel: w673 -> [w738]
          tunnel: w672 -> [w737]
          tunnel: w595 -> [w752]
          shift-right: [w753] -> w666
          shift-left: w671 -> [w754]
          tunnel: w592 -> [w748]
          tunnel: w591 -> [w742]
          shift-right: [w739] -> _
          shift-left: w629 -> [w743]
          stop <- w755 stop-if-true
          n378 = Less?(x=w743, y=w748) -> (x < y?=w746:bool)
          n379 = Less?(x=w743, y=w742) -> (x < y?=w744:bool)
          n380 = call "Bis zum nächsten Vielfachen warten13"("Count(mSec)"=u32 100 ("Zu wartende ms")) -> ()  [unwired: 1 out]
          n381 = global read "GVMethodenwechsel.vi" "Methodenwechsel?"() -> (w757:bool)
          n382 = global read "gvbooleschRT.vi" "global stop RT"() -> (w758:bool)
          n383 = local read "veränderte Methode benutzen"() -> (w756:bool)
          n384 = Compound Arithmetic op=OR(w758, w757, w756) -> (w755:bool)
          n385 = global read "GVZeitenZyklen.vi" "Big Ben, Methodenzeit, Zykluszeit0, Zykluszeit1, Zykluszeit2A, Zykluszeit2B"() -> (w750:dbl[])
          n386 = Index Array(array=w750, index=3 ("Index")) -> (element=w739:dbl)
          n387 = Greater Or Equal?(x=w739, y=w748) -> (x >= y?=w747:bool)
          n388 = Greater Or Equal?(x=w739, y=w742) -> (x >= y?=w745:bool)
          n389 = And(x=w745, y=w744) -> (x .and. y?=w741:bool)
          n390 = And(x=w747, y=w746) -> (x .and. y?=w736:bool)
          n391 = Or(x=w736, y=w741) -> (x .or. y?=w740:bool)
          n392 = And(x=w752, y=w740) -> (x .and. y?=w751:bool)
          n393 = case shown="True" w751 {
            tunnel: w754 -> [w760 w761]
            tunnel: [w760 w765] -> w753
            tunnel: w738 -> [_ w764]
            tunnel: w737 -> [_ w763]
            tunnel: w736 -> [_ w762]
            frame False {
            }
            frame True {
              n394 = call "MSDateienSchicken12-15.vi"("MSNummer"=w761, "MSa?"=w762, "Dateipfad:fromcriordy"=w763, "Dateipfad:fromcriocmd"=w764) -> ()  [unwired: 1 in]
              n395 = Increment(x=w761) -> (x+1=w765:i32)
            }
          }
        }
      }
      n396 = while {
        stop <- w1023 stop-if-true
        w1017 = 10.0
        n397 = call "Warten2"("Count(mSec)"=u32 1000) -> ()  [unwired: 1 out]
        n398 = global read "gvbooleschRT.vi" "global stop RT"() -> (w1023:bool)
        n399 = global read "GVTrapsMachs.vi" "Traps/Machs"() -> (w1013:dbl[])
        n400 = global read "GVAIs.vi" "AIs"() -> (w1014:dbl[])
        n401 = for {
          N: 9 -> [_]
          shift-right: [w1026] -> w1020
          shift-left: w1014 -> [w1027]
          shift-right: [w1024] -> w1018
          shift-left: w1013 -> [w1025]
          n402 = flat-sequence {
            tunnel: w1027 -> [w1034]
            tunnel: [w1033] -> w1026
            tunnel: w1025 -> [w1032]
            tunnel: [w1031] -> w1024
            frame #0 {
              n403 = call "Warten28"("Count(mSec)"=u32 100) -> ()  [unwired: 1 out]
            }
            frame #1 {
              n404 = global read "GVAIs.vi" "AIs"() -> (w1030:dbl[])
              n405 = Add(x=w1034, y=w1030) -> (x+y=w1033:dbl[])
              n406 = global read "GVTrapsMachs.vi" "Traps/Machs"() -> (w1029:dbl[])
              n407 = Add(x=w1029, y=w1032) -> (x+y=w1031:dbl[])
            }
          }
        }
        n408 = Divide(x=w1020, y=w1017) -> (x/y=w1019:dbl[])
        n409 = Divide(x=w1018, y=w1017) -> (x/y=w1016:dbl[])
        n410 = Build Array (concatenate)(w1019, w1016) -> (w1015:dbl[])
        n411 = global write "GVHK1Hz.vi" "Mod1Mod2Mod3/AITrapsMachs1Hz"(w1015) -> ()
      }
      n412 = Add Array Elements(numeric array=w293) -> (sum=w362:i32)
      n413 = Index Array(array=w293, index #1=0 ("Index"), index #2=1 ("Index")) -> (element #1=w373:i32, element #2=w371:i32)
      n414 = case shown="True" TRUE ("ECDSpeichern") {
        frame False {
        }
        frame True {
          w489 = dbl[] []
          n415 = global read "GVaktuelleTDMS.vi" "aktuelleTDMS-DateiECD1"() -> (w490:refnum<k34>)
          n416 = while {
            shift-right: [w502] -> _
            shift-left: w489 -> [w506]
            shift-right: [w495] -> _
            shift-left: w489 -> [w499]
            shift-right: [w501] -> _
            shift-left: w490 -> [w504]
            tunnel: w489 -> [w498]
            shift-right: [w491] -> _
            shift-left: errorcluster {"status"=FALSE, "code"=0, "source"=""} ("error IO") -> [w492]
            stop <- w511 stop-if-true
            n417 = call "Bis zum nächsten Vielfachen warten3"("Count(mSec)"=u32 500) -> ()  [unwired: 1 out]
            n418 = global read "GVECDs.vi" "ECD1MW"() -> (w505:dbl[])
            n419 = global read "GVECDs.vi" "ECD2MW"() -> (w496:dbl[])
            n420 = global read "gvbooleschRT.vi" "global stop RT"() -> (w511:bool)
            n421 = Build Array (concatenate)(w506, w505) -> (w503:dbl[])
            n422 = Build Array (concatenate)(w499, w496) -> (w500:dbl[])
            n423 = global read "GVaktuelleTDMS.vi" "aktuelleTDMS-DateiECD1"() -> (w501:refnum<k34>)
            n424 = global read "GVaktuelleTDMS.vi" "aktuelleTDMS-DateiECD2"() -> (w509:refnum<k34>)
            n425 = Equal?(x=w504, y=w501) -> (x = y?=w497:bool)
            n426 = TDMS Write(0:w501, 7:"ECD1", 9:w505, 11:w492) -> (15:w494:errorcluster)  [unwired: 2 in, 3 out]
            n427 = TDMS Write(0:w509, 7:"ECD2", 9:w496, 11:w492) -> (15:w493:errorcluster)  [unwired: 2 in, 3 out]
            n428 = Select(t=w503, s=w497, f=w498) -> (s? t:f=w502:dbl[])
            n429 = Select(t=w500, s=w497, f=w498) -> (s? t:f=w495:dbl[])
            n430 = global write "GVChroms.vi" "ECD1Chrom"(w502) -> ()
            n431 = global write "GVChroms.vi" "ECD2Chrom"(w495) -> ()
            n432 = Merge Errors(w494, w493) -> (w491:errorcluster)
            "TDMSwriteECD" <- w491
          }
        }
      }
      n433 = while {
        shift-right: [w395] -> _
        shift-left: w303 -> [w397]
        shift-right: [w394] -> _
        shift-left: w303 -> [w396]
        stop <- w399 stop-if-true
        n434 = call "Bis zum nächsten Vielfachen warten"("Count(mSec)"=u32 100) -> ()  [unwired: 1 out]
        n435 = case shown="True" "An/Aus" {
          tunnel: w397 -> [w401 w417]
          tunnel: w396 -> [w400 w416]
          tunnel: [w401 w410] -> w395
          tunnel: [w400 w409] -> w394
          frame False {
          }
          frame True {
            w413 = dbl[] [] ("t")
            n436 = global read "GVMWHorst.vi" "MWHorst"() -> (w406:dbl[])
            n437 = global read "GVTrapsMachs.vi" "Traps/Machs"() -> (w407:dbl[])
            n438 = Build Array (concatenate)(w407, w406) -> (w405:dbl[])
            n439 = Index Array(array=w405, index="dargestellte Größe 3") -> (element=w418:dbl)
            n440 = Build Array (concatenate)(w417, w418) -> (w411:dbl[])
            n441 = Select(t=w413, s="TafelWischen!", f=w411) -> (s? t:f=w410:dbl[])
            n442 = global read "GVZeitenZyklen.vi" "Big Ben, Methodenzeit, Zykluszeit0, Zykluszeit1, Zykluszeit2A, Zykluszeit2B"() -> (w404:dbl[])
            n443 = Index Array(array=w404, index=1 ("Index")) -> (element=w402:dbl)
            n444 = Build Array (concatenate)(w416, w402) -> (w412:dbl[])
            n445 = Select(t=w413, s="TafelWischen!", f=w412) -> (s? t:f=w409:dbl[])
            n446 = Bundle(w412, w411) -> (→"schnelleAnzeige":cluster{dbl[], dbl[]})  [unwired: 1 in]
          }
        }
        n447 = global read "gvbooleschRT.vi" "global stop RT"() -> (w399:bool)
      }
      n448 = Split 1D Array(array=w352, index=w373) -> (first subarray=w377:dbl[], second subarray=w381:dbl[])
      n449 = Split 1D Array(array=w294, index=w373) -> (first subarray=w380:string[], second subarray=w382:string[])
      n450 = Split 1D Array(array=w351, index=w373) -> (first subarray=w370:string[], second subarray=w372:string[])
      n451 = Initialize Array(-1.0 ("Element"), w362) -> (w349:dbl[])
      n452 = case shown="True" TRUE {
        tunnel: w343 -> [_ w521]
        tunnel: w341 -> [_ w520]
        tunnel: w340 -> [_ w519]
        tunnel: w335 -> [_ w518]
        tunnel: w334 -> [_ w517]
        frame False {
        }
        frame True {
          w512 = errorcluster {"status"=FALSE, "code"=0, "source"=""} ("error out TDMSopen")
          n453 = while {
            shift-right: [w526] -> w516
            shift-left: w518 -> [w528]
            shift-right: [w537] -> w515
            shift-left: w517 -> [w530]
            shift-right: [w532] -> _
            shift-left: w521 -> [w538]
            tunnel: w519 -> [w534]
            tunnel: w520 -> [w535]
            shift-right: [w525] -> w514
            shift-left: w512 -> [w523]
            shift-right: [w524] -> w513
            shift-left: w512 -> [w522]
            stop <- w540 stop-if-true
            n454 = call "Bis zum nächsten Vielfachen warten5"("Count(mSec)"=u32 500) -> ()  [unwired: 1 out]
            n455 = local read "Methode"() -> (w536:i32)
            n456 = global read "gvbooleschRT.vi" "global stop RT"() -> (w540:bool)
            n457 = global read "GVZeitenZyklen.vi" "ZyklusNummernGesamt"() -> (w527:i32[])
            n458 = Index Array(array=w527, index=1 ("Index")) -> (element=w532:i32)
            n459 = Greater?(x=w532, y=w538) -> (0:w531:bool)
            n460 = Select(t=w530, s=w531, f=w528) -> (s? t:f=w529:refnum<k34>)
            n461 = call "AktuelleTDMS.vi"("AktuelleTDMS"=w528, "error in TDMSopen"=w523, "Dateiordner"=w535, "NächsteTDMS"=w530, "NeuerZyklus?"=w531, "Methodennummer"=w536, "Zyklnumges"=w532, "error in TDMSclose"=w522, "Dateiname"=w534) -> ("AktuelleTDMS"=w526:refnum<k34>, "error out TDMSopen"=w525:errorcluster, "error out TDMSclose"=w524:errorcluster, "NächsteTDMS"=w537:refnum<k34>)  [unwired: 3 in]
            "TDMSopenHK" <- w525
            "TDMScloseHK" <- w524
            n462 = global write "GVaktuelleTDMS.vi" "aktuelleTDMS-DateiHK"(w529) -> ()
          }
          n463 = TDMS Close(8:w514, 11:w516) -> ()  [unwired: 2 out]
          n464 = TDMS Close(8:w513, 11:w515) -> ()  [unwired: 2 out]
        }
      }
      n465 = case shown="True" TRUE {
        tunnel: w343 -> [_ w449]
        tunnel: w339 -> [_ w448]
        tunnel: w338 -> [_ w447]
        tunnel: w337 -> [_ w446]
        tunnel: w336 -> [_ w445]
        tunnel: w333 -> [_ w444]
        tunnel: w332 -> [_ w443]
        tunnel: w331 -> [_ w442]
        tunnel: w330 -> [_ w441]
        frame False {
        }
        frame True {
          w434 = errorcluster {"status"=FALSE, "code"=0, "source"=""} ("error out TDMSopen")
          n466 = while {
            shift-right: [w473] -> w440
            shift-left: w444 -> [w475]
            shift-right: [w483] -> w439
            shift-left: w443 -> [w477]
            shift-right: [w481] -> _
            shift-left: w449 -> [w484]
            tunnel: w448 -> [w480]
            tunnel: w446 -> [w479]
            shift-right: [w472] -> w435
            shift-left: w434 -> [w470]
            shift-right: [w471] -> w436
            shift-left: w434 -> [w469]
            stop <- w486 stop-if-true
            n467 = call "Bis zum nächsten Vielfachen warten4"("Count(mSec)"=u32 500) -> ()  [unwired: 1 out]
            n468 = local read "Methode"() -> (w482:i32)
            n469 = global read "gvbooleschRT.vi" "global stop RT"() -> (w486:bool)
            n470 = global read "GVZeitenZyklen.vi" "ZyklusNummernGesamt"() -> (w474:i32[])
            n471 = Index Array(array=w474, index=2 ("Index")) -> (element=w481:i32)
            n472 = Greater?(x=w481, y=w484) -> (0:w478:bool)
            n473 = Select(t=w477, s=w478, f=w475) -> (s? t:f=w476:refnum<k34>)
            n474 = call "AktuelleTDMS.vi"("AktuelleTDMS"=w475, "error in TDMSopen"=w470, "Dateiordner"=w480, "NächsteTDMS"=w477, "NeuerZyklus?"=w478, "Methodennummer"=w482, "Zyklnumges"=w481, "error in TDMSclose"=w469, "Dateiname"=w479) -> ("AktuelleTDMS"=w473:refnum<k34>, "error out TDMSopen"=w472:errorcluster, "error out TDMSclose"=w471:errorcluster, "NächsteTDMS"=w483:refnum<k34>)  [unwired: 3 in]
            "TDMSopenECD1" <- w472
            "TDMScloseECD1" <- w471
            n475 = global write "GVaktuelleTDMS.vi" "aktuelleTDMS-DateiECD1"(w476) -> ()
          }
          n476 = while {
            shift-right: [w463] -> w438
            shift-left: w442 -> [w455]
            shift-right: [w464] -> w437
            shift-left: w441 -> [w457]
            shift-right: [w461] -> _
            shift-left: w449 -> [w465]
            tunnel: w447 -> [w460]
            tunnel: w445 -> [w459]
            shift-right: [w453] -> _
            shift-left: w434 -> [w451]
            shift-right: [w452] -> _
            shift-left: w434 -> [w450]
            stop <- w467 stop-if-true
            n477 = call "Bis zum nächsten Vielfachen warten6"("Count(mSec)"=u32 500) -> ()  [unwired: 1 out]
            n478 = local read "Methode"() -> (w462:i32)
            n479 = global read "gvbooleschRT.vi" "global stop RT"() -> (w467:bool)
            n480 = global read "GVZeitenZyklen.vi" "ZyklusNummernGesamt"() -> (w454:i32[])
            n481 = Index Array(array=w454, index=3 ("Index")) -> (element=w461:i32)
            n482 = Greater?(x=w461, y=w465) -> (0:w458:bool)
            n483 = Select(t=w457, s=w458, f=w455) -> (s? t:f=w456:refnum<k34>)
            n484 = call "AktuelleTDMS.vi"("AktuelleTDMS"=w455, "error in TDMSopen"=w451, "Dateiordner"=w460, "NächsteTDMS"=w457, "NeuerZyklus?"=w458, "Methodennummer"=w462, "Zyklnumges"=w461, "error in TDMSclose"=w450, "Dateiname"=w459) -> ("AktuelleTDMS"=w463:refnum<k34>, "error out TDMSopen"=w453:errorcluster, "error out TDMSclose"=w452:errorcluster, "NächsteTDMS"=w464:refnum<k34>)  [unwired: 3 in]
            "TDMSopenECD2" <- w453
            "TDMScloseECD2" <- w452
            n485 = global write "GVaktuelleTDMS.vi" "aktuelleTDMS-DateiECD2"(w456) -> ()
          }
          n486 = TDMS Close(8:w435, 11:w440) -> ()  [unwired: 2 out]
          n487 = TDMS Close(8:w436, 11:w439) -> ()  [unwired: 2 out]
          n488 = TDMS Close(11:w438) -> ()  [unwired: 1 in, 2 out]
          n489 = TDMS Close(11:w437) -> ()  [unwired: 1 in, 2 out]
        }
      }
      n490 = Split 1D Array(array=w382, index=w371) -> (first subarray=w379:string[], second subarray=w378:string[])
      n491 = Split 1D Array(array=w381, index=w371) -> (first subarray=w376:dbl[], second subarray=w375:dbl[])
      n492 = Split 1D Array(array=w372, index=w371) -> (first subarray=w369:string[], second subarray=w368:string[])
      n493 = Bundle(w380, w379, w378, w377, w376, w375) -> (w374:T16)  [unwired: 1 in]
      n494 = Bundle(w370, w369, w368) -> (w367:cluster{string[], string[], string[]})  [unwired: 1 in]
      n495 = Bundle(w366, w366, w366) -> (w365:cluster{i32, i32, i32})  [unwired: 1 in]
      n496 = Initialize Array("x", 8 ("Dimension")) -> (w306:string[])
      n497 = case shown="True" TRUE ("SerielleKomm.") {
        tunnel: bool[] [TRUE, TRUE, TRUE, TRUE, TRUE, TRUE, TRUE, TRUE] -> [_ _]
        tunnel: w306 -> [_ _]
        tunnel: w374 -> [_ w427]
        tunnel: w373 -> [_ _]
        tunnel: w371 -> [_ _]
        tunnel: w367 -> [_ w424]
        tunnel: w365 -> [_ _]
        tunnel: w364 -> [_ _]
        tunnel: w352 -> [_ _]
        tunnel: w350 -> [_ _]
        tunnel: w349 -> [_ _]
        tunnel: w348 -> [_ w429]
        tunnel: w329 -> [_ _]
        tunnel: w292 -> [_ w423]
        frame False {
        }
        frame True {
          n498 = Unbundle(w424) -> (w422:string[])  [unwired: 2 out]
          n499 = Unbundle(w427) -> (w425:string[], w426:dbl[])  [unwired: 4 out]
          n500 = while {
            stop <- w433 stop-if-true
            n501 = global write "GVRefStrom.vi" "RefStromECD2"("RefStromECD2") -> ()
            n502 = global write "GVRefStrom.vi" "RefStromECD1"("RefStromECD1") -> ()
            n503 = global read "gvbooleschRT.vi" "global stop RT"() -> (w433:bool)
            n504 = call "Bis zum nächsten Vielfachen warten17"("Count(mSec)"=u32 500) -> ()  [unwired: 1 out]
          }
          n505 = Array Size(array=w422) -> (size(s)=w421:i32)
          n506 = Initialize Array("xxx", w421) -> (w419:string[])
          n507 = call "Seriell-ECD.vi"("FPGA-VI-Referenz"=w429, "SPvorgebenMod2"=w425, "MWabfragenMod2"=w422, "MWAntwortMod2"=w423, "FaktorMod2"=w426, "SPquittieren"=w419) -> ("Fehler"=→"SerielleKomm.":errorcluster)  [unwired: 9 in]
        }
      }
    }
    frame #2 {
      n508 = xnode "Element lesen/schreiben"("FPGA-VI-Referenz (Eingang)"=w1042, "global stop"=TRUE) -> ("FPGA-VI-Referenz (Ausgang)"=w1041:refnum<k20>)  [unwired: 1 in, 1 out]
      n509 = xnode "Close FPGA VI Reference"("FPGA-VI-Referenz (Eingang)"=w1041) -> ()  [unwired: 1 in, 1 out]
    }
    frame #3 {
    }
    frame #4 {
    }
  }
